vi "HEWH Dispense Schedule.vi"(0 "Core HEWH Data Input":T1={"Scan Rate Adjust"=0.0, "Draw Count"=0, "Test Patten Setup"={"Total Gallons Schedule"=[10.0, 10.0, 10.0, 10.0], "PRAT/RLT Sequence"=[{"Sequence #"=1.0, "Cycles"=35, "Mode Setting"="", "Flow Rate (GPM)"=0.0, "Temperature (F)"=0.0, "Reset Timer"=FALSE, "Use Temp Decline Method"=FALSE, "Terminate Condition"=enum."C1-Terminate Draw @ Gallon Mark", "Condition Value #1"=1.0, "UE"=FALSE, "LE"=FALSE, "Comp"=FALSE, "Fan"=FALSE, "Test End Time (Sec)"=0.0, "Purge Until Cutout"=FALSE, "Start Conditions"=enum."Heat Source Cutout", "Condition Value #2"=0.0, "Remove Power"=FALSE, "Time"=0.0, "Check Special Cond."=enum."SC1-Do Nothing", "Condition#"=enum."C1", "Draw Flags"=enum."N/A", "Data Processing Delay (FHD 15sec, UEF 5 Sec)"=0.0, "Test Complete"=FALSE, "User Setpoint"=0.0, "Tank Setpoint"=0.0}, {"Sequence #"=2.0, "Cycles"=15, "Mode Setting"="", "Flow Rate (GPM)"=0.0, "Temperature (F)"=0.0, "Reset Timer"=FALSE, "Use Temp Decline Method"=FALSE, "Terminate Condition"=enum."C1-Terminate Draw @ Gallon Mark", "Condition Value #1"=1.0, "UE"=FALSE, "LE"=FALSE, "Comp"=FALSE, "Fan"=FALSE, "Test End Time (Sec)"=0.0, "Purge Until Cutout"=FALSE, "Start Conditions"=enum."Heat Source Cutout", "Condition Value #2"=0.0, "Remove Power"=FALSE, "Time"=0.0, "Check Special Cond."=enum."SC1-Do Nothing", "Condition#"=enum."C1", "Draw Flags"=enum."N/A", "Data Processing Delay (FHD 15sec, UEF 5 Sec)"=0.0, "Test Complete"=FALSE, "User Setpoint"=0.0, "Tank Setpoint"=0.0}, {"Sequence #"=3.0, "Cycles"=35, "Mode Setting"="", "Flow Rate (GPM)"=0.0, "Temperature (F)"=0.0, "Reset Timer"=FALSE, "Use Temp Decline Method"=FALSE, "Terminate Condition"=enum."C1-Terminate Draw @ Gallon Mark", "Condition Value #1"=2.0, "UE"=FALSE, "LE"=FALSE, "Comp"=FALSE, "Fan"=FALSE, "Test End Time (Sec)"=0.0, "Purge Until Cutout"=FALSE, "Start Conditions"=enum."Heat Source Cutout", "Condition Value #2"=0.0, "Remove Power"=FALSE, "Time"=0.0, "Check Special Cond."=enum."SC1-Do Nothing", "Condition#"=enum."C1", "Draw Flags"=enum."N/A", "Data Processing Delay (FHD 15sec, UEF 5 Sec)"=0.0, "Test Complete"=FALSE, "User Setpoint"=0.0, "Tank Setpoint"=0.0}, {"Sequence #"=4.0, "Cycles"=15, "Mode Setting"="", "Flow Rate (GPM)"=0.0, "Temperature (F)"=0.0, "Reset Timer"=FALSE, "Use Temp Decline Method"=FALSE, "Terminate Condition"=enum."C1-Terminate Draw @ Gallon Mark", "Condition Value #1"=2.0, "UE"=FALSE, "LE"=FALSE, "Comp"=FALSE, "Fan"=FALSE, "Test End Time (Sec)"=0.0, "Purge Until Cutout"=FALSE, "Start Conditions"=enum."Heat Source Cutout", "Condition Value #2"=0.0, "Remove Power"=FALSE, "Time"=0.0, "Check Special Cond."=enum."SC1-Do Nothing", "Condition#"=enum."C1", "Draw Flags"=enum."N/A", "Data Processing Delay (FHD 15sec, UEF 5 Sec)"=0.0, "Test Complete"=FALSE, "User Setpoint"=0.0, "Tank Setpoint"=0.0}, {"Sequence #"=5.0, "Cycles"=35, "Mode Setting"="", "Flow Rate (GPM)"=0.0, "Temperature (F)"=0.0, "Reset Timer"=FALSE, "Use Temp Decline Method"=FALSE, "Terminate Condition"=enum."C1-Terminate Draw @ Gallon Mark", "Condition Value #1"=0.0, "UE"=FALSE, "LE"=FALSE, "Comp"=FALSE, "Fan"=FALSE, "Test End Time (Sec)"=0.0, "Purge Until Cutout"=FALSE, "Start Conditions"=enum."Heat Source Cutout", "Condition Value #2"=0.0, "Remove Power"=FALSE, "Time"=0.0, "Check Special Cond."=enum."SC1-Do Nothing", "Condition#"=enum."C1", "Draw Flags"=enum."N/A", "Data Processing Delay (FHD 15sec, UEF 5 Sec)"=0.0, "Test Complete"=FALSE, "User Setpoint"=0.0, "Tank Setpoint"=0.0}, {"Sequence #"=6.0, "Cycles"=15, "Mode Setting"="", "Flow Rate (GPM)"=0.0, "Temperature (F)"=0.0, "Reset Timer"=FALSE, "Use Temp Decline Method"=FALSE, "Terminate Condition"=enum."C1-Terminate Draw @ Gallon Mark", "Condition Value #1"=0.0, "UE"=FALSE, "LE"=FALSE, "Comp"=FALSE, "Fan"=FALSE, "Test End Time (Sec)"=0.0, "Purge Until Cutout"=FALSE, "Start Conditions"=enum."Heat Source Cutout", "Condition Value #2"=0.0, "Remove Power"=FALSE, "Time"=0.0, "Check Special Cond."=enum."SC1-Do Nothing", "Condition#"=enum."C1", "Draw Flags"=enum."N/A", "Data Processing Delay (FHD 15sec, UEF 5 Sec)"=0.0, "Test Complete"=FALSE, "User Setpoint"=0.0, "Tank Setpoint"=0.0}, {"Sequence #"=7.0, "Cycles"=35, "Mode Setting"="", "Flow Rate (GPM)"=0.0, "Temperature (F)"=0.0, "Reset Timer"=FALSE, "Use Temp Decline Method"=FALSE, "Terminate Condition"=enum."C1-Terminate Draw @ Gallon Mark", "Condition Value #1"=1.0, "UE"=FALSE, "LE"=FALSE, "Comp"=FALSE, "Fan"=FALSE, "Test End Time (Sec)"=0.0, "Purge Until Cutout"=FALSE, "Start Conditions"=enum."Heat Source Cutout", "Condition Value #2"=0.0, "Remove Power"=FALSE, "Time"=0.0, "Check Special Cond."=enum."SC1-Do Nothing", "Condition#"=enum."C1", "Draw Flags"=enum."N/A", "Data Processing Delay (FHD 15sec, UEF 5 Sec)"=0.0, "Test Complete"=FALSE, "User Setpoint"=0.0, "Tank Setpoint"=0.0}, {"Sequence #"=8.0, "Cycles"=15, "Mode Setting"="", "Flow Rate (GPM)"=0.0, "Temperature (F)"=0.0, "Reset Timer"=FALSE, "Use Temp Decline Method"=FALSE, "Terminate Condition"=enum."C1-Terminate Draw @ Gallon Mark", "Condition Value #1"=1.0, "UE"=FALSE, "LE"=FALSE, "Comp"=FALSE, "Fan"=FALSE, "Test End Time (Sec)"=0.0, "Purge Until Cutout"=FALSE, "Start Conditions"=enum."Heat Source Cutout", "Condition Value #2"=0.0, "Remove Power"=FALSE, "Time"=0.0, "Check Special Cond."=enum."SC1-Do Nothing", "Condition#"=enum."C1", "Draw Flags"=enum."N/A", "Data Processing Delay (FHD 15sec, UEF 5 Sec)"=0.0, "Test Complete"=FALSE, "User Setpoint"=0.0, "Tank Setpoint"=0.0}], "Current Sequence Index"=0}, "HEWH Specific DAQ"={"HEWH Data"={"HEWH Standard"={"Voltage (Volts)"=0.0, "Current (Amps)"=0.0, "Power (Watts)"=0.0, "WattHours (Wh)"=0.0, "TC Tree (AVG)"=0.0, "Flow Rate (GPM)"=0.0, "Gallons (Gal)"=0.0, "RTD Out (Deg F)"=0.0, "RTD In (Deg F)"=0.0, "RTD Amb (Deg F)"=0.0, "TC Down"=0.0, "UE Event Lead"=0, "LE Event Lead"=0, "TC Tree Array"=[]}, "PRAT"={"Power (Watts) A"=4192.0, "Power (Watts) B"=4192.0, "Power (Watts) C"=4192.0, "Power (Watts) D"=4192.0, "TC1"=0.0, "TC2"=0.0, "TC3"=0.0, "TC4"=0.0, "WattHours (Wh) A"=4192.0, "WattHours (Wh) B"=4192.0, "WattHours (Wh) C"=4192.0, "WattHours (Wh) D"=4192.0, "Ambient"=0.0, "Extra Temp"=0.0}, "Additional Power Data"={"Vthd"=236.2, "Frequency (Hz)"=236.2, "Apparent Power (VA)"=236.2, "Power Factor"=236.2, "Current Crest Factor"=236.2, "Voltage Crest Factor"=236.2, "Integration Time (sec)"=236.2}}, "Flow Valve % Open"=0.0, "Power State"={"UE"=FALSE, "LE"=FALSE, "COMP"=FALSE, "FANS"=FALSE}, "Power Analyzer"=enum."APLUS", "Flow Valve uA Output"=0, "Gallons Start (Gal)"=0.0}, "Test Output Data"={"PreDraw Data Table"=[], "Data Table"=[], "MW100 TC Headers"=[]}, "Calc and Calibration"={"Mean SD Var Max Min Array"=[], "Draw Statistics (DBL)"=[], "Calibration Coefficients DBL"=[], "Start Gallons"=0.0, "Starting Temp Decline"=0.0, "K-Factor (Temperature)"=0.0, "All Draw Stats"=[], "RTD Terminate Value"=0.0, "K-Factor (Flow)"=0.0, "Intellifaucet Type"="", "Thermal Stabil Array"=[], "Gas Thermal Stabil Complete"=FALSE, "Therm Reset Cmpt 1"=FALSE, "Therm Reset Cmpt 2"=FALSE, "Last Flow Rate (Therm)"=0.0, "State"=enum."State 0", "Gas Thermal Time"=0.0, "Target Rate (Thermal)"=0.0, "Thermal - Final"=[], "State5 Gal Water"=0.0, "State 5 Gal Gas"=0.0, "Intellif Open < 1"=0.0, "Intellif Open < 1.7"=0.0, "Intellif Open < 2.2"=0.0, "Intellif Open > 2.2"=0.0}, "Current Draw Time"=0.0, "LV Program"=enum."HEWH", "Station ID"=enum."A", "Current Cond"=enum."N/A", "Test Complete"=FALSE, "ANSI Rate"={"Array 1"=[], "Array 3"=[], "Array 2"=[], "Start ANSI"=FALSE, "ANSI Start Time"=0.0, "Restart ANSI"=FALSE, "15 Min ANSI Avg (BTU/hr)"=0.0, "20 Min ANSI Avg (BTU/hr)"=0.0, "25 Min ANSI Avg (BTU/hr)"=0.0, "Absolute Pressure"=0.0, "Gas Temperature"=0.0, "Volumetric Flow Rate"=0.0, "Mass Flow Rate"=0.0, "Array 4"=[], "Array 5"=[], "Gas Rate"=0.0, "15 Min Pres Avg (PSIA)"=0.0, "20 Min Pres Avg (PSIA)"=0.0, "25 Min Pres Avg (PSIA)"=0.0, "15 Min Temp Avg (°F) "=0.0, "20 Min Temp Avg (°F)"=0.0, "25 Min Temp Avg (°F)"=0.0, "15 Min Uncorrected Avg (CFH)"=0.0, "20 Min Uncorrected Avg (CFH)"=0.0, "25 Min Uncorrected Avg (CFH)"=0.0, "15 Min Corrected Avg (SCFH)"=0.0, "20 Min Corrected Avg (SCFH)"=0.0, "25 Min Corrected Avg (SCFH)"=0.0, "15 Min Complete"=FALSE, "20 Min Complete"=FALSE, "25 Min Complete"=FALSE, "Heating Value (BTU/ft³)"=0.0, "CO CO2 15 Min"=[], "CO CO2 20 Min"=[], "CO CO2 25 Min"=[], "CO CO2 Real Time"=[]}, "Gas Measurment Data"={"Absolute Pressure"=0.0, "Gauge/Diff. Pressure"=0.0, "Barometric Pressure"=0.0, "Temperature"=0.0, "Volumetric Flow"=0.0, "Mass Flow"=0.0, "Setpoint"=0.0, "Valve Drive"=0.0, "Totalizer"=0.0, "[hr]"=0.0, "[min]"=0.0, "[sec]"=0.0, "Totalizer Average Flow"=0.0, "Totalizer Peak Flow"=0.0, "Gas selected"=""}, "Module 4 Relay Status"={"INTELLIFAUCET TEMP(T)/FLOW(F) (CH 041)"=FALSE, "INTELLIFAUCET READY (CH 042)"=FALSE, "INTELLIFAUCET START (CH 043)"=FALSE, "INTELLIFAUCET STOP (CH 044)"=FALSE, "MAIN POWER RELAY (CH 047)"=FALSE, "NOT USED (CH 045)"=FALSE, "NOT USED (CH 046)"=FALSE, "PURGE VALVE RELAY (CH 048)"=FALSE, "OUTLET VALVE RELAY (CH 049)"=FALSE, "INLET VALVE RELAY (CH 050)"=FALSE, "Intellifaucet (% Open)"=0.0, "Proportioning Valve (%Open)"=0.0, "Intellifaucet Temp Setpoint (F)"=0.0}} {"Test Patten Setup"."PRAT/RLT Sequence"."Time" format="%<%H:%M:%S>t"; "Test Patten Setup"."Total Gallons Schedule" format="%.2f"}, 5 "Hide PreDraw Tab":bool, 11 "error in (no error)":errorcluster) -> (4 "Core HEWH Data Input Out":T1={"Scan Rate Adjust"=1000.0, "Draw Count"=0, "Test Patten Setup"={"Total Gallons Schedule"=[10.72, 10.72, 10.72, 10.72, 10.72, 10.72], "PRAT/RLT Sequence"=[{"Sequence #"=1.0, "Cycles"=35, "Mode Setting"="", "Flow Rate (GPM)"=0.0, "Temperature (F)"=0.0, "Reset Timer"=FALSE, "Use Temp Decline Method"=FALSE, "Terminate Condition"=enum."C1-Terminate Draw @ Gallon Mark", "Condition Value #1"=1.0, "UE"=FALSE, "LE"=FALSE, "Comp"=FALSE, "Fan"=FALSE, "Test End Time (Sec)"=0.0, "Purge Until Cutout"=FALSE, "Start Conditions"=enum."Heat Source Cutout", "Condition Value #2"=0.0, "Remove Power"=FALSE, "Time"=0.0, "Check Special Cond."=enum."SC1-Do Nothing", "Condition#"=enum."C1", "Draw Flags"=enum."N/A", "Data Processing Delay (FHD 15sec, UEF 5 Sec)"=0.0, "Test Complete"=FALSE, "User Setpoint"=0.0, "Tank Setpoint"=0.0}, {"Sequence #"=2.0, "Cycles"=15, "Mode Setting"="", "Flow Rate (GPM)"=0.0, "Temperature (F)"=0.0, "Reset Timer"=FALSE, "Use Temp Decline Method"=FALSE, "Terminate Condition"=enum."C1-Terminate Draw @ Gallon Mark", "Condition Value #1"=1.0, "UE"=FALSE, "LE"=FALSE, "Comp"=FALSE, "Fan"=FALSE, "Test End Time (Sec)"=0.0, "Purge Until Cutout"=FALSE, "Start Conditions"=enum."Heat Source Cutout", "Condition Value #2"=0.0, "Remove Power"=FALSE, "Time"=0.0, "Check Special Cond."=enum."SC1-Do Nothing", "Condition#"=enum."C1", "Draw Flags"=enum."N/A", "Data Processing Delay (FHD 15sec, UEF 5 Sec)"=0.0, "Test Complete"=FALSE, "User Setpoint"=0.0, "Tank Setpoint"=0.0}, {"Sequence #"=3.0, "Cycles"=35, "Mode Setting"="", "Flow Rate (GPM)"=0.0, "Temperature (F)"=0.0, "Reset Timer"=FALSE, "Use Temp Decline Method"=FALSE, "Terminate Condition"=enum."C1-Terminate Draw @ Gallon Mark", "Condition Value #1"=2.0, "UE"=FALSE, "LE"=FALSE, "Comp"=FALSE, "Fan"=FALSE, "Test End Time (Sec)"=0.0, "Purge Until Cutout"=FALSE, "Start Conditions"=enum."Heat Source Cutout", "Condition Value #2"=0.0, "Remove Power"=FALSE, "Time"=0.0, "Check Special Cond."=enum."SC1-Do Nothing", "Condition#"=enum."C1", "Draw Flags"=enum."N/A", "Data Processing Delay (FHD 15sec, UEF 5 Sec)"=0.0, "Test Complete"=FALSE, "User Setpoint"=0.0, "Tank Setpoint"=0.0}, {"Sequence #"=4.0, "Cycles"=15, "Mode Setting"="", "Flow Rate (GPM)"=0.0, "Temperature (F)"=0.0, "Reset Timer"=FALSE, "Use Temp Decline Method"=FALSE, "Terminate Condition"=enum."C1-Terminate Draw @ Gallon Mark", "Condition Value #1"=2.0, "UE"=FALSE, "LE"=FALSE, "Comp"=FALSE, "Fan"=FALSE, "Test End Time (Sec)"=0.0, "Purge Until Cutout"=FALSE, "Start Conditions"=enum."Heat Source Cutout", "Condition Value #2"=0.0, "Remove Power"=FALSE, "Time"=0.0, "Check Special Cond."=enum."SC1-Do Nothing", "Condition#"=enum."C1", "Draw Flags"=enum."N/A", "Data Processing Delay (FHD 15sec, UEF 5 Sec)"=0.0, "Test Complete"=FALSE, "User Setpoint"=0.0, "Tank Setpoint"=0.0}, {"Sequence #"=5.0, "Cycles"=35, "Mode Setting"="", "Flow Rate (GPM)"=0.0, "Temperature (F)"=0.0, "Reset Timer"=FALSE, "Use Temp Decline Method"=FALSE, "Terminate Condition"=enum."C1-Terminate Draw @ Gallon Mark", "Condition Value #1"=0.0, "UE"=FALSE, "LE"=FALSE, "Comp"=FALSE, "Fan"=FALSE, "Test End Time (Sec)"=0.0, "Purge Until Cutout"=FALSE, "Start Conditions"=enum."Heat Source Cutout", "Condition Value #2"=0.0, "Remove Power"=FALSE, "Time"=0.0, "Check Special Cond."=enum."SC1-Do Nothing", "Condition#"=enum."C1", "Draw Flags"=enum."N/A", "Data Processing Delay (FHD 15sec, UEF 5 Sec)"=0.0, "Test Complete"=FALSE, "User Setpoint"=0.0, "Tank Setpoint"=0.0}, {"Sequence #"=6.0, "Cycles"=15, "Mode Setting"="", "Flow Rate (GPM)"=0.0, "Temperature (F)"=0.0, "Reset Timer"=FALSE, "Use Temp Decline Method"=FALSE, "Terminate Condition"=enum."C1-Terminate Draw @ Gallon Mark", "Condition Value #1"=0.0, "UE"=FALSE, "LE"=FALSE, "Comp"=FALSE, "Fan"=FALSE, "Test End Time (Sec)"=0.0, "Purge Until Cutout"=FALSE, "Start Conditions"=enum."Heat Source Cutout", "Condition Value #2"=0.0, "Remove Power"=FALSE, "Time"=0.0, "Check Special Cond."=enum."SC1-Do Nothing", "Condition#"=enum."C1", "Draw Flags"=enum."N/A", "Data Processing Delay (FHD 15sec, UEF 5 Sec)"=0.0, "Test Complete"=FALSE, "User Setpoint"=0.0, "Tank Setpoint"=0.0}, {"Sequence #"=7.0, "Cycles"=35, "Mode Setting"="", "Flow Rate (GPM)"=0.0, "Temperature (F)"=0.0, "Reset Timer"=FALSE, "Use Temp Decline Method"=FALSE, "Terminate Condition"=enum."C1-Terminate Draw @ Gallon Mark", "Condition Value #1"=1.0, "UE"=FALSE, "LE"=FALSE, "Comp"=FALSE, "Fan"=FALSE, "Test End Time (Sec)"=0.0, "Purge Until Cutout"=FALSE, "Start Conditions"=enum."Heat Source Cutout", "Condition Value #2"=0.0, "Remove Power"=FALSE, "Time"=0.0, "Check Special Cond."=enum."SC1-Do Nothing", "Condition#"=enum."C1", "Draw Flags"=enum."N/A", "Data Processing Delay (FHD 15sec, UEF 5 Sec)"=0.0, "Test Complete"=FALSE, "User Setpoint"=0.0, "Tank Setpoint"=0.0}, {"Sequence #"=8.0, "Cycles"=15, "Mode Setting"="", "Flow Rate (GPM)"=0.0, "Temperature (F)"=0.0, "Reset Timer"=FALSE, "Use Temp Decline Method"=FALSE, "Terminate Condition"=enum."C1-Terminate Draw @ Gallon Mark", "Condition Value #1"=1.0, "UE"=FALSE, "LE"=FALSE, "Comp"=FALSE, "Fan"=FALSE, "Test End Time (Sec)"=0.0, "Purge Until Cutout"=FALSE, "Start Conditions"=enum."Heat Source Cutout", "Condition Value #2"=0.0, "Remove Power"=FALSE, "Time"=0.0, "Check Special Cond."=enum."SC1-Do Nothing", "Condition#"=enum."C1", "Draw Flags"=enum."N/A", "Data Processing Delay (FHD 15sec, UEF 5 Sec)"=0.0, "Test Complete"=FALSE, "User Setpoint"=0.0, "Tank Setpoint"=0.0}], "Current Sequence Index"=0}, "HEWH Specific DAQ"={"HEWH Data"={"HEWH Standard"={"Voltage (Volts)"=-1.0, "Current (Amps)"=-1.0, "Power (Watts)"=-1.0, "WattHours (Wh)"=-1.0, "TC Tree (AVG)"=0.0, "Flow Rate (GPM)"=0.0, "Gallons (Gal)"=0.0, "RTD Out (Deg F)"=0.0, "RTD In (Deg F)"=0.0, "RTD Amb (Deg F)"=0.0, "TC Down"=0.0, "UE Event Lead"=0, "LE Event Lead"=0, "TC Tree Array"=[]}, "PRAT"={"Power (Watts) A"=4192.0, "Power (Watts) B"=4192.0, "Power (Watts) C"=4192.0, "Power (Watts) D"=4192.0, "TC1"=0.0, "TC2"=0.0, "TC3"=0.0, "TC4"=0.0, "WattHours (Wh) A"=4192.0, "WattHours (Wh) B"=4192.0, "WattHours (Wh) C"=4192.0, "WattHours (Wh) D"=4192.0, "Ambient"=0.0, "Extra Temp"=0.0}, "Additional Power Data"={"Vthd"=236.2, "Frequency (Hz)"=236.2, "Apparent Power (VA)"=236.2, "Power Factor"=236.2, "Current Crest Factor"=236.2, "Voltage Crest Factor"=236.2, "Integration Time (sec)"=236.2}}, "Flow Valve % Open"=0.0, "Power State"={"UE"=FALSE, "LE"=FALSE, "COMP"=FALSE, "FANS"=FALSE}, "Power Analyzer"=enum."APLUS", "Flow Valve uA Output"=0, "Gallons Start (Gal)"=0.0}, "Test Output Data"={"PreDraw Data Table"=[], "Data Table"=[], "MW100 TC Headers"=[]}, "Calc and Calibration"={"Mean SD Var Max Min Array"=[], "Draw Statistics (DBL)"=[], "Calibration Coefficients DBL"=[], "Start Gallons"=0.0, "Starting Temp Decline"=1000.0, "K-Factor (Temperature)"=0.0, "All Draw Stats"=[], "RTD Terminate Value"=0.0, "K-Factor (Flow)"=0.0, "Intellifaucet Type"="", "Thermal Stabil Array"=[], "Gas Thermal Stabil Complete"=FALSE, "Therm Reset Cmpt 1"=FALSE, "Therm Reset Cmpt 2"=FALSE, "Last Flow Rate (Therm)"=0.0, "State"=enum."State 0", "Gas Thermal Time"=0.0, "Target Rate (Thermal)"=0.0, "Thermal - Final"=[], "State5 Gal Water"=0.0, "State 5 Gal Gas"=0.0, "Intellif Open < 1"=0.0, "Intellif Open < 1.7"=0.0, "Intellif Open < 2.2"=0.0, "Intellif Open > 2.2"=0.0}, "Current Draw Time"=0.0, "LV Program"=enum."HEWH", "Station ID"=enum."A", "Current Cond"=enum."N/A", "Test Complete"=FALSE, "ANSI Rate"={"Array 1"=[], "Array 3"=[], "Array 2"=[], "Start ANSI"=FALSE, "ANSI Start Time"=0.0, "Restart ANSI"=FALSE, "15 Min ANSI Avg (BTU/hr)"=0.0, "20 Min ANSI Avg (BTU/hr)"=0.0, "25 Min ANSI Avg (BTU/hr)"=0.0, "Absolute Pressure"=0.0, "Gas Temperature"=0.0, "Volumetric Flow Rate"=0.0, "Mass Flow Rate"=0.0, "Array 4"=[], "Array 5"=[], "Gas Rate"=0.0, "15 Min Pres Avg (PSIA)"=0.0, "20 Min Pres Avg (PSIA)"=0.0, "25 Min Pres Avg (PSIA)"=0.0, "15 Min Temp Avg (°F) "=0.0, "20 Min Temp Avg (°F)"=0.0, "25 Min Temp Avg (°F)"=0.0, "15 Min Uncorrected Avg (CFH)"=0.0, "20 Min Uncorrected Avg (CFH)"=0.0, "25 Min Uncorrected Avg (CFH)"=0.0, "15 Min Corrected Avg (SCFH)"=0.0, "20 Min Corrected Avg (SCFH)"=0.0, "25 Min Corrected Avg (SCFH)"=0.0, "15 Min Complete"=FALSE, "20 Min Complete"=FALSE, "25 Min Complete"=FALSE, "Heating Value (BTU/ft³)"=0.0, "CO CO2 15 Min"=[], "CO CO2 20 Min"=[], "CO CO2 25 Min"=[], "CO CO2 Real Time"=[]}, "Gas Measurment Data"={"Absolute Pressure"=0.0, "Gauge/Diff. Pressure"=0.0, "Barometric Pressure"=0.0, "Temperature"=0.0, "Volumetric Flow"=0.0, "Mass Flow"=0.0, "Setpoint"=0.0, "Valve Drive"=0.0, "Totalizer"=0.0, "[hr]"=0.0, "[min]"=0.0, "[sec]"=0.0, "Totalizer Average Flow"=0.0, "Totalizer Peak Flow"=0.0, "Gas selected"=""}, "Module 4 Relay Status"={"INTELLIFAUCET TEMP(T)/FLOW(F) (CH 041)"=FALSE, "INTELLIFAUCET READY (CH 042)"=FALSE, "INTELLIFAUCET START (CH 043)"=FALSE, "INTELLIFAUCET STOP (CH 044)"=FALSE, "MAIN POWER RELAY (CH 047)"=FALSE, "NOT USED (CH 045)"=FALSE, "NOT USED (CH 046)"=FALSE, "PURGE VALVE RELAY (CH 048)"=FALSE, "OUTLET VALVE RELAY (CH 049)"=FALSE, "INLET VALVE RELAY (CH 050)"=FALSE, "Intellifaucet (% Open)"=0.0, "Proportioning Valve (%Open)"=0.0, "Intellifaucet Temp Setpoint (F)"=0.0}} {"Test Patten Setup"."PRAT/RLT Sequence"."Time" format="%<%H:%M:%S>t"; "Test Patten Setup"."Total Gallons Schedule" format="%.2f"}, 15 "error out":errorcluster)   [LabVIEW 2019]
uses:
  Type Definitions/HEWH PreDraw.ctl
  Type Definitions/HEWH Draw Pattern Setup.ctl
  Type Definitions/HEWH Power Elements.ctl
  Type Definitions/HEWH Power Data.ctl
  Utility/Type Definitions/UTILITY Power Analyzer.ctl
  Type Definitions/HEWH Output Information.ctl
  Utility/Save File/File Setup (Public)/Type Definition/Save File DOE LabView Program.ctl
  Utility/Save File/File Setup.lvlib
  Custom Instrument Control/MW100/Type Definitions/Station ID Selector.ctl
  Utility/Save File/File Setup (Public)/Type Definition/Save File HEWH Heating Control Mode.ctl
  Type Definitions/PRAT Test.ctl
  Type Definitions/HEWH Calc and Calibration.ctl
  Draw Water Specific/Type Definitions/Terminate Draw Conditions.ctl
  Type Definitions/HEWH Start Conditions.ctl
  Type Definitions/HEWH Specific DAQ.ctl
  Draw Water Specific/Type Definitions/Check Special Condtions.ctl
  Type Definitions/HEWH Draw Flag ENUM.ctl
  Draw Water Specific/Type Definitions/HEWH Special Condition Check.ctl
  Range/Type Definitions/RANGE ANSI Rate.ctl
  Drivers/Alicat Gas Meter Driver/Sub-VIs/Data Cluster.ctl
  Custom Instrument Control/MW100/Type Definitions/HEWH Module 4 Relay Status.ctl
panel:
  in  "Tab Control":enum32{"Input", "Diagnostics"}(tab)
  out "Display and Exit":bool
  out "PreDraw\nPattern":dbl[][](array[numeric])
  in  "Draw Pattern Setup Tab":T20(tab)
  in  "Populate Older":bool
  in  "Populate Low Usage":bool
  in  "Populate Medium Usage":bool
  in  "Populate High Usage":bool
  in  "Pattern Setup":dbl[][](array[numeric])
  in  "High Usage":bool
  in  "Medium Usage":bool
  in  "Low Usage":bool
  in  "Older":bool
  out "Description":string="Pre-Draw Setup"
  out "Description 1":string="Pre-Draw Setup"
  in  "Total Gallons (1)":dbl=10.72
  in  "Flow Rate (GPM 1)":dbl=3.0
  in  "Incoming Water Temperature (1)":dbl=58.0
  out "Description 4":string="OR"
  in  "Any Heat (1)":bool
  in  "Any Heat (2)":bool
  in  "Any Heat (3)":bool
  out "Description 2":string="Pre-Draw Setup"
  in  "Total Gallons (2)":dbl=10.72
  in  "Flow Rate (GPM 2)":dbl=3.0
  in  "Incoming Water Temperature (2)":dbl=58.0
  out "Description 3":string="Pre-Draw Setup"
  in  "Total Gallons (3)":dbl=10.72
  in  "Flow Rate (GPM 3)":dbl=3.0
  in  "Incoming Water Temperature (3)":dbl=58.0
  out "Description 5":string="OR"
  out "Description 6":string="OR"
  in  "PreDraw Enum":T21=enum.""
  in  "stop":bool
  # "Draw Patten Setup"
  # "Totalizer Timer"
  # "Draw Pattern Setup (24 Hour)"
  # "Totalizer Timer"
  # "Draw Pattern Setup (24 Hour)"
  # "Dispense Times\n(Hour)"
  # "Dispense Times\n(Minutes)"
  # "Dispense Times\n(Seconds)"
  # "Total Gallons"
  # "Flow Rate\n(GPM)"
  # "Incoming Water\n Temperature"
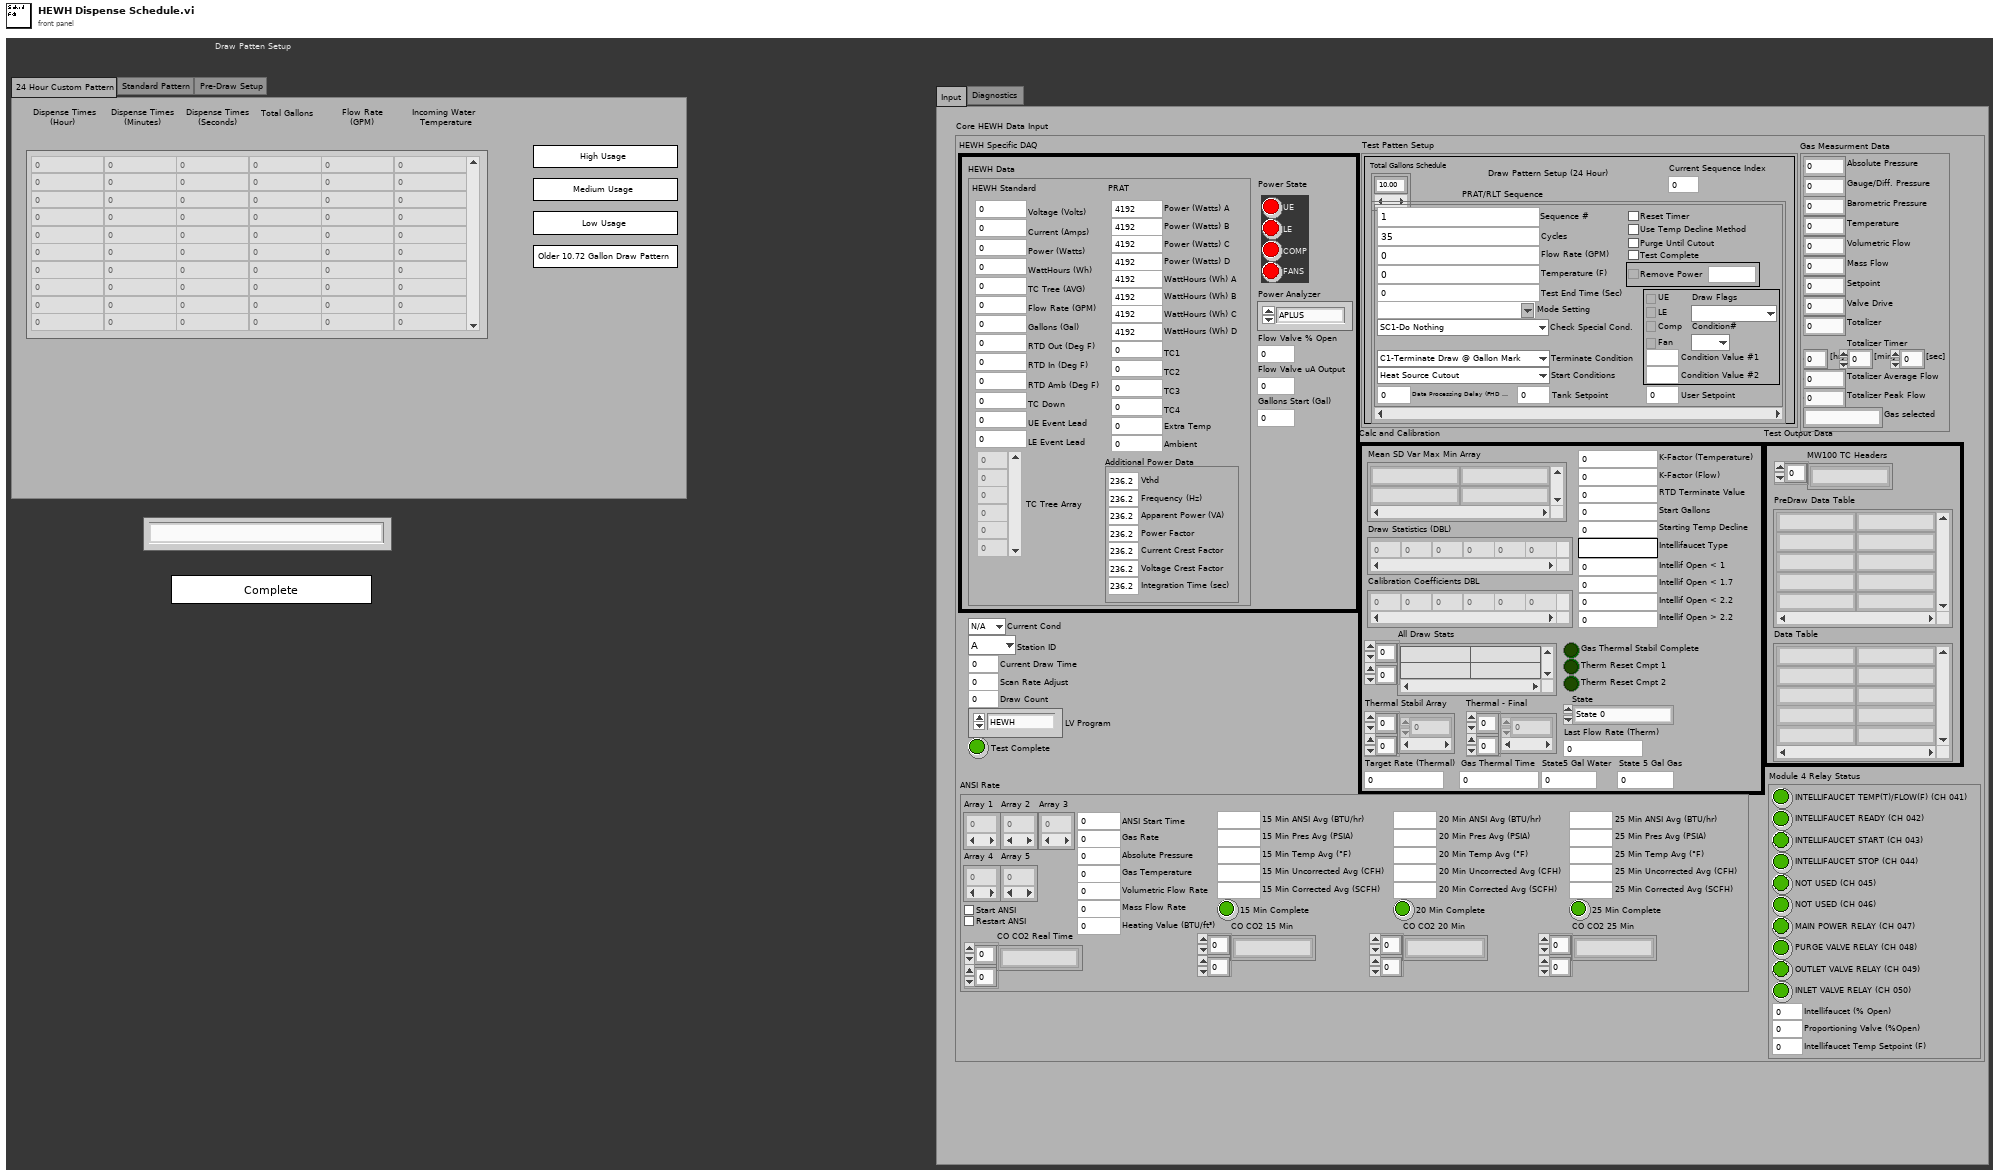
[diagram p1: front panel]
types:
  T1 = typedef "HEWH Output Information.ctl" = cluster{"Scan Rate Adjust":dbl, "Draw Count":i32, "Test Patten Setup":T2, "HEWH Specific DAQ":T10, "Test Output Data":cluster{"PreDraw Data Table":string[][], "Data Table":string[][], "MW100 TC Headers":string[]}, "Calc and Calibration":T14, "Current Draw Time":dbl, "LV Program":T15, "Station ID":T16, "Current Cond":T8, "Test Complete":bool, "ANSI Rate":T17, "Gas Measurment Data":T18, "Module 4 Relay Status":T19}
  T2 = typedef "HEWH Draw Pattern Setup.ctl" = cluster{"Total Gallons Schedule":dbl[], "PRAT/RLT Sequence":T3[], "Current Sequence Index":i32}
  T3 = typedef "PRAT Test.ctl" = cluster{"Sequence #":dbl, "Cycles":i32, "Mode Setting":T4, "Flow Rate (GPM)":dbl, "Temperature (F)":dbl, "Reset Timer":bool, "Use Temp Decline Method":bool, "Terminate Condition":T5, "Condition Value #1":dbl, "UE":bool, "LE":bool, "Comp":bool, "Fan":bool, "Test End Time (Sec)":dbl, "Purge Until Cutout":bool, "Start Conditions":T6, "Condition Value #2":dbl, "Remove Power":bool, "Time":dbl, "Check Special Cond.":T7, "Condition#":T8, "Draw Flags":T9, "Data Processing Delay (FHD 15sec, UEF 5 Sec)":dbl, "Test Complete":bool, "User Setpoint":dbl, "Tank Setpoint":dbl}
  T4 = typedef "File Setup.lvlib/Save File HEWH Heating Control Mode.ctl" = string
  T5 = typedef "Terminate Draw Conditions.ctl" = enum16{"C1-Terminate Draw @ Gallon Mark", "C2-Special Last Draw (HU Test)", "C3-RTD Out <=", "C4-Mean Tank Temp <=", "C5-Decrease RTD Out (Deg F)", "C6-Time (Seconds)", "C7-Until Any Heat Source", "C8-Specific Heat Source", "C9-Do Nothing", "C10-Inlet Outlet RTD Temp Delta"}
  T6 = typedef "HEWH Start Conditions.ctl" = enum16{"Heat Source Cutout", "At Time (Seconds)", "Every X (Seconds)", "T2 >= X° Below Setpoint", "Seconds From Complete", "Wait for LE & Comp Cutout", "Wait for Comp Cutout", "Wait for LE Cutout", "Wait for UE Cutout", "Start Immediately"}
  T7 = typedef "Check Special Condtions.ctl" = enum16{"SC1-Do Nothing", "SC2-Check Heat Source (On-C2/Off-C1)", "SC3-Check Skip Condition", "SC4-Check Heat Source ON/Fail", "SC5-Keep Draw Valves Open", "SC6-Skip Purge"}
  T8 = typedef "HEWH Special Condition Check.ctl" = enum16{"N/A", "C1", "C2", "Reset/Fail", "Skip Draw Sequence"}
  T9 = typedef "HEWH Draw Flag ENUM.ctl" = enum16{"N/A", "None(0)", "Sml(1)", "Med(2)", "SmlMed(3)", "Lrg(4)", "SmlLrg(5)", "MedLrg(6)", "SmlMedLrg(7)"}
  T10 = typedef "HEWH Specific DAQ.ctl" = cluster{"HEWH Data":T11, "Flow Valve % Open":dbl, "Power State":T12, "Power Analyzer":T13, "Flow Valve uA Output":i32, "Gallons Start (Gal)":dbl}
  T11 = typedef "HEWH Power Data.ctl" = cluster{"HEWH Standard":cluster{"Voltage (Volts)":dbl, "Current (Amps)":dbl, "Power (Watts)":dbl, "WattHours (Wh)":dbl, "TC Tree (AVG)":dbl, "Flow Rate (GPM)":dbl, "Gallons (Gal)":dbl, "RTD Out (Deg F)":dbl, "RTD In (Deg F)":dbl, "RTD Amb (Deg F)":dbl, "TC Down":dbl, "UE Event Lead":i32, "LE Event Lead":i32, "TC Tree Array":dbl[]}, "PRAT":cluster{"Power (Watts) A":dbl, "Power (Watts) B":dbl, "Power (Watts) C":dbl, "Power (Watts) D":dbl, "TC1":dbl, "TC2":dbl, "TC3":dbl, "TC4":dbl, "WattHours (Wh) A":dbl, "WattHours (Wh) B":dbl, "WattHours (Wh) C":dbl, "WattHours (Wh) D":dbl, "Ambient":dbl, "Extra Temp":dbl}, "Additional Power Data":cluster{"Vthd":dbl, "Frequency (Hz)":dbl, "Apparent Power (VA)":dbl, "Power Factor":dbl, "Current Crest Factor":dbl, "Voltage Crest Factor":dbl, "Integration Time (sec)":dbl}}
  T12 = typedef "HEWH Power Elements.ctl" = cluster{"UE":bool, "LE":bool, "COMP":bool, "FANS":bool}
  T13 = typedef "UTILITY Power Analyzer.ctl" = enum16{"", "APLUS", "WT210", "WT500", "WT300", "OSI", "Debug", "WT230", "WT300_1", "WT300_2"}
  T14 = typedef "HEWH Calc and Calibration.ctl" = cluster{"Mean SD Var Max Min Array":string[][], "Draw Statistics (DBL)":dbl[][], "Calibration Coefficients DBL":dbl[][], "Start Gallons":dbl, "Starting Temp Decline":dbl, "K-Factor (Temperature)":dbl, "All Draw Stats":string[][], "RTD Terminate Value":dbl, "K-Factor (Flow)":dbl, "Intellifaucet Type":string, "Thermal Stabil Array":dbl[][], "Gas Thermal Stabil Complete":bool, "Therm Reset Cmpt 1":bool, "Therm Reset Cmpt 2":bool, "Last Flow Rate (Therm)":dbl, "State":enum16{"State 0", "State 1", "State 2", "State 3", "State 4", "State 5", "State 6"}, "Gas Thermal Time":dbl, "Target Rate (Thermal)":dbl, "Thermal - Final":dbl[][], "State5 Gal Water":dbl, "State 5 Gal Gas":dbl, "Intellif Open < 1":dbl, "Intellif Open < 1.7":dbl, "Intellif Open < 2.2":dbl, "Intellif Open > 2.2":dbl}
  T15 = typedef "File Setup.lvlib/Save File DOE LabView Program.ctl" = enum16{"No Name Found", "DOE Stand", "Dishwasher Kitchen", "Portable Stand", "HEWH", "Dryer", "Dryer WILT", "HCC", "PRAT", "HEWH RLT", "Refrigeration", "Gas Water Heater"}
  T16 = typedef "Station ID Selector.ctl" = enum16{"", "A", "B", "C", "D", "Global"}
  T17 = typedef "RANGE ANSI Rate.ctl" = cluster{"Array 1":dbl[], "Array 3":dbl[], "Array 2":dbl[], "Start ANSI":bool, "ANSI Start Time":dbl, "Restart ANSI":bool, "15 Min ANSI Avg (BTU/hr)":dbl, "20 Min ANSI Avg (BTU/hr)":dbl, "25 Min ANSI Avg (BTU/hr)":dbl, "Absolute Pressure":dbl, "Gas Temperature":dbl, "Volumetric Flow Rate":dbl, "Mass Flow Rate":dbl, "Array 4":dbl[], "Array 5":dbl[], "Gas Rate":dbl, "15 Min Pres Avg (PSIA)":dbl, "20 Min Pres Avg (PSIA)":dbl, "25 Min Pres Avg (PSIA)":dbl, "15 Min Temp Avg (°F) ":dbl, "20 Min Temp Avg (°F)":dbl, "25 Min Temp Avg (°F)":dbl, "15 Min Uncorrected Avg (CFH)":dbl, "20 Min Uncorrected Avg (CFH)":dbl, "25 Min Uncorrected Avg (CFH)":dbl, "15 Min Corrected Avg (SCFH)":dbl, "20 Min Corrected Avg (SCFH)":dbl, "25 Min Corrected Avg (SCFH)":dbl, "15 Min Complete":bool, "20 Min Complete":bool, "25 Min Complete":bool, "Heating Value (BTU/ft³)":dbl, "CO CO2 15 Min":string[][], "CO CO2 20 Min":string[][], "CO CO2 25 Min":string[][], "CO CO2 Real Time":string[][]}
  T18 = typedef "Data Cluster.ctl" = cluster{"Absolute Pressure":dbl, "Gauge/Diff. Pressure":dbl, "Barometric Pressure":dbl, "Temperature":dbl, "Volumetric Flow":dbl, "Mass Flow":dbl, "Setpoint":dbl, "Valve Drive":dbl, "Totalizer":dbl, "[hr]":dbl, "[min]":dbl, "[sec]":dbl, "Totalizer Average Flow":dbl, "Totalizer Peak Flow":dbl, "Gas selected":string}
  T19 = typedef "HEWH Module 4 Relay Status.ctl" = cluster{"INTELLIFAUCET TEMP(T)/FLOW(F) (CH 041)":bool, "INTELLIFAUCET READY (CH 042)":bool, "INTELLIFAUCET START (CH 043)":bool, "INTELLIFAUCET STOP (CH 044)":bool, "MAIN POWER RELAY (CH 047)":bool, "NOT USED (CH 045)":bool, "NOT USED (CH 046)":bool, "PURGE VALVE RELAY (CH 048)":bool, "OUTLET VALVE RELAY (CH 049)":bool, "INLET VALVE RELAY (CH 050)":bool, "Intellifaucet (% Open)":dbl, "Proportioning Valve (%Open)":dbl, "Intellifaucet Temp Setpoint (F)":dbl}
  T20 = enum32{"24 Hour Custom Pattern", "Standard Pattern", "Pre-Draw Setup"}
  T21 = typedef "HEWH PreDraw.ctl" = enum16{"Zero Pre-Draws", "One Pre- Draws", "Two Pre-Draws", "Three Pre-Draws", ""}
  T22 = enum32{"invalid app kind", "Development System", "Run Time System", "Student Edition", "Embedded LabVIEW", "Evaluation", "Custom"}
  T23 = enum32{"Invalid", "Standard", "Closed", "Hidden", "Minimized", "Maximized"}
  T24 = cluster{"Core":cluster{"Current VI Reference":refnum<vi>, "Close Panel on Exit?":bool}, "Pattern Setup":dbl[][], "Core HEWH Data Input":T1, "PreDraw Enum":T21, "Any Heat (1)":bool, "Any Heat (2)":bool, "Any Heat (3)":bool}
  T25 = cluster{"Current VI Reference":refnum<vi>, "Close Panel on Exit?":bool}
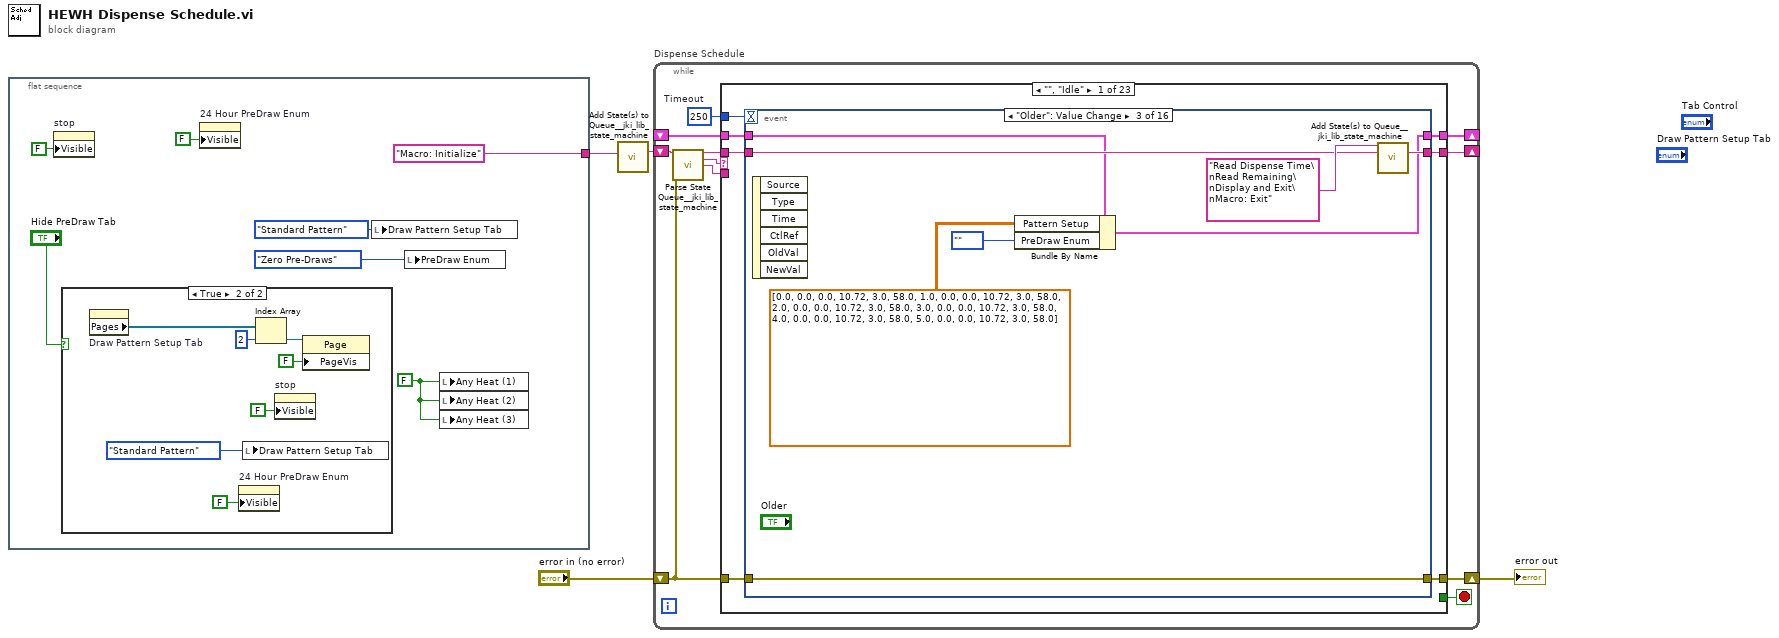
[diagram p0: block diagram]
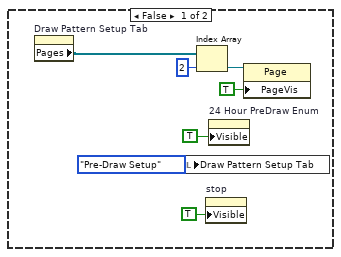
[diagram p2: hidden frame]
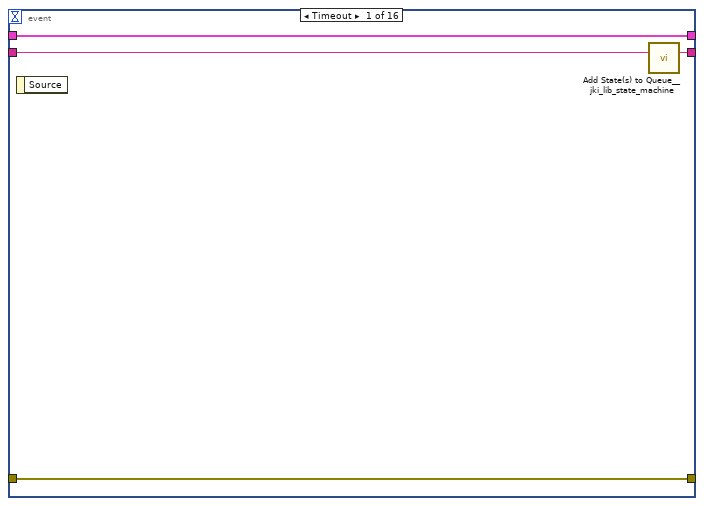
[diagram p3: hidden frame]
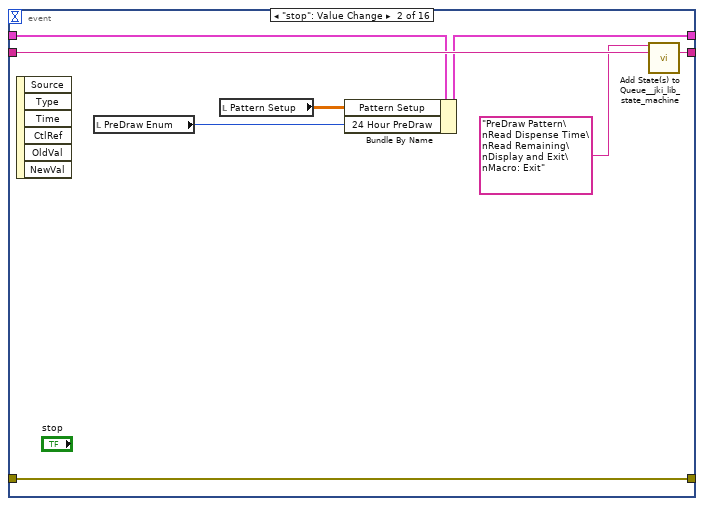
[diagram p4: hidden frame]
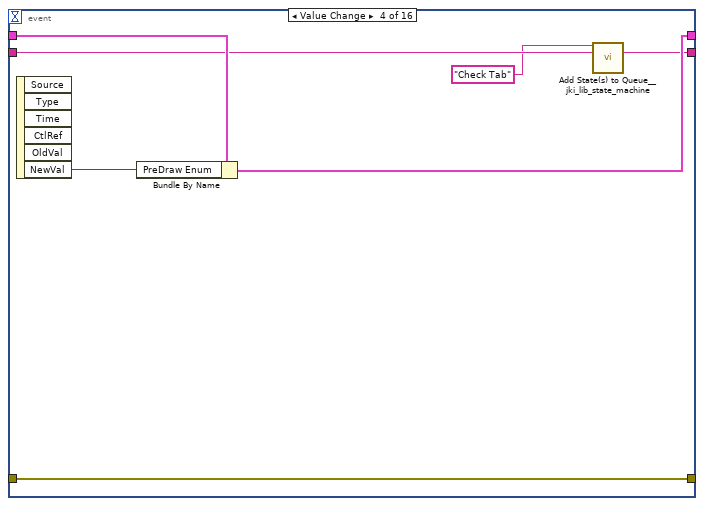
[diagram p5: hidden frame]
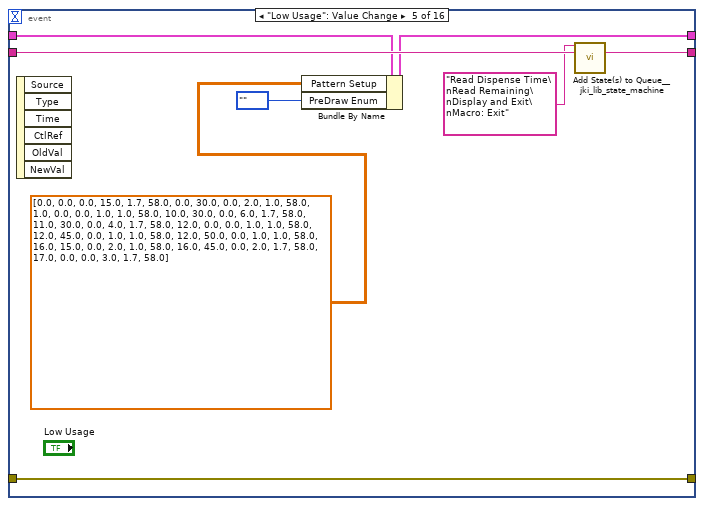
[diagram p6: hidden frame]
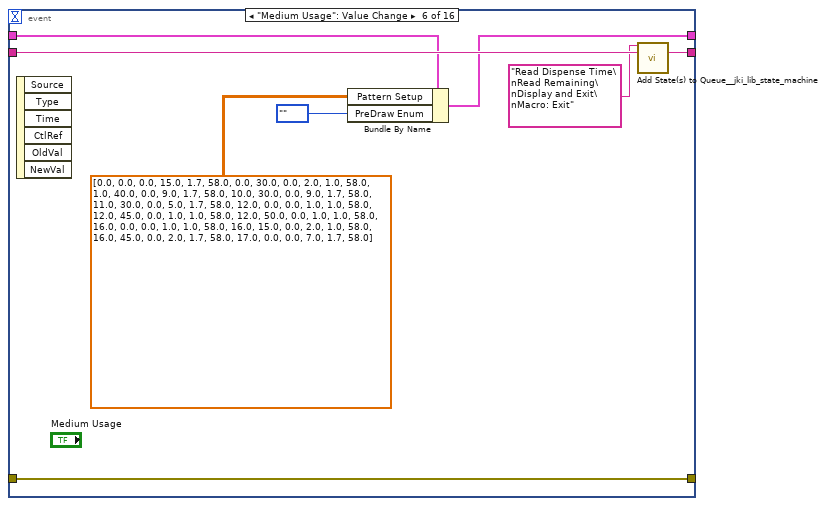
[diagram p7: hidden frame]
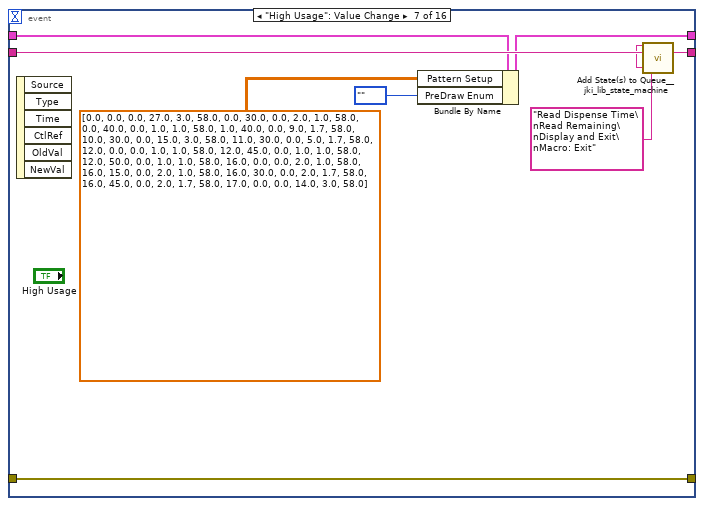
[diagram p8: hidden frame]
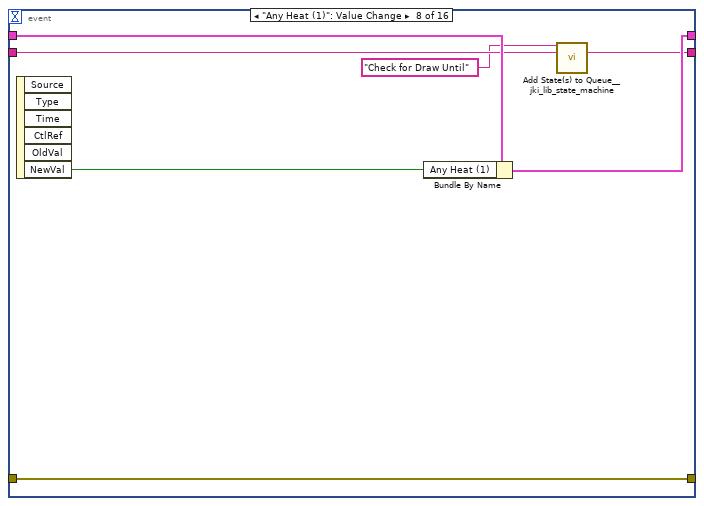
[diagram p9: hidden frame]
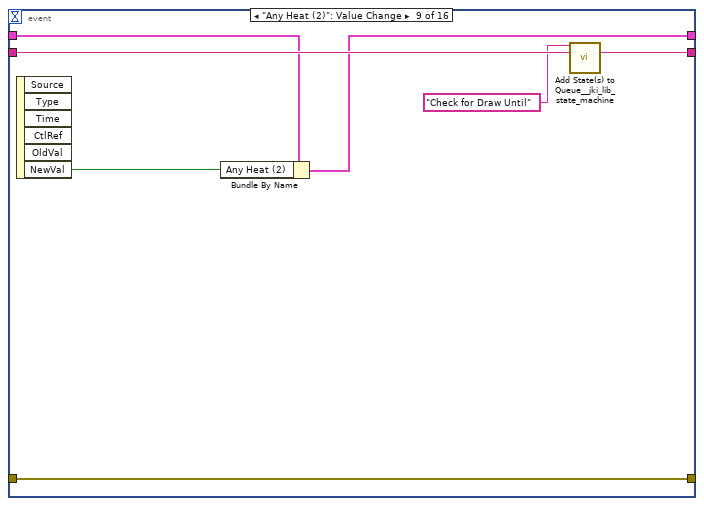
[diagram p10: hidden frame]
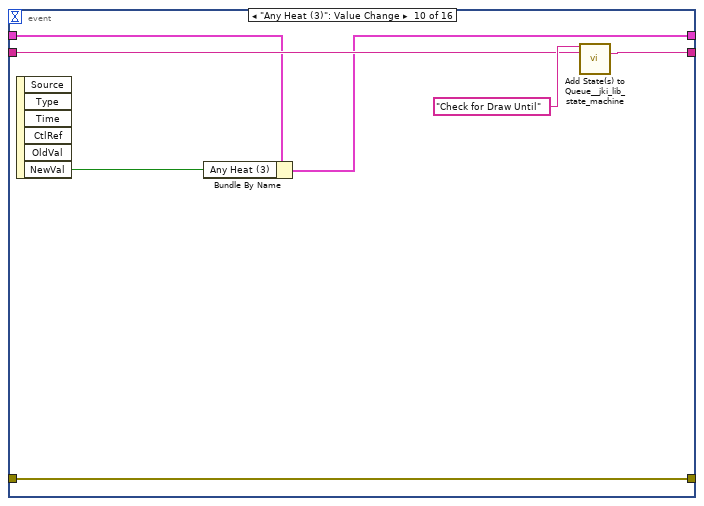
[diagram p11: hidden frame]
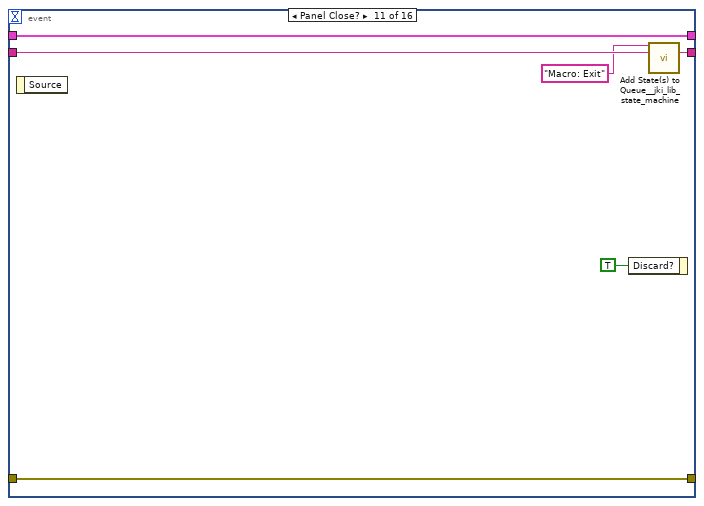
[diagram p12: hidden frame]
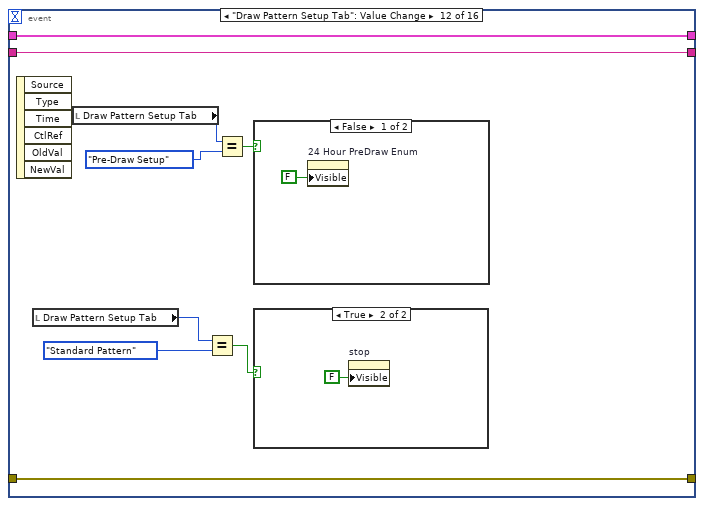
[diagram p13: hidden frame]
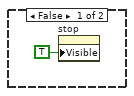
[diagram p14: hidden frame]
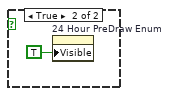
[diagram p15: hidden frame]
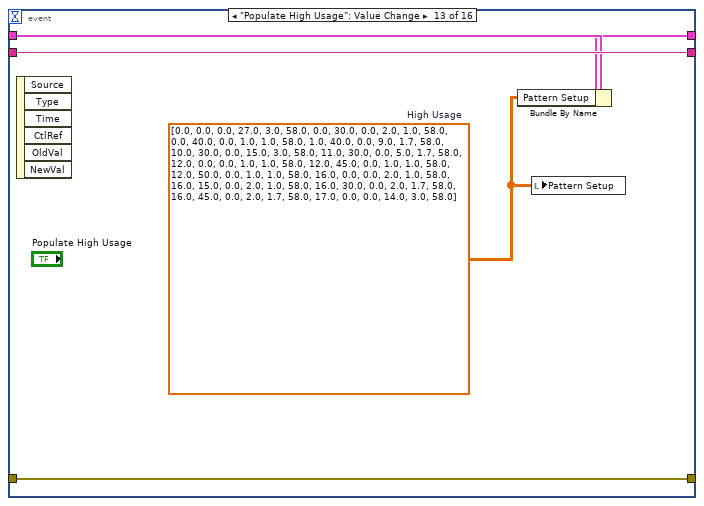
[diagram p16: hidden frame]
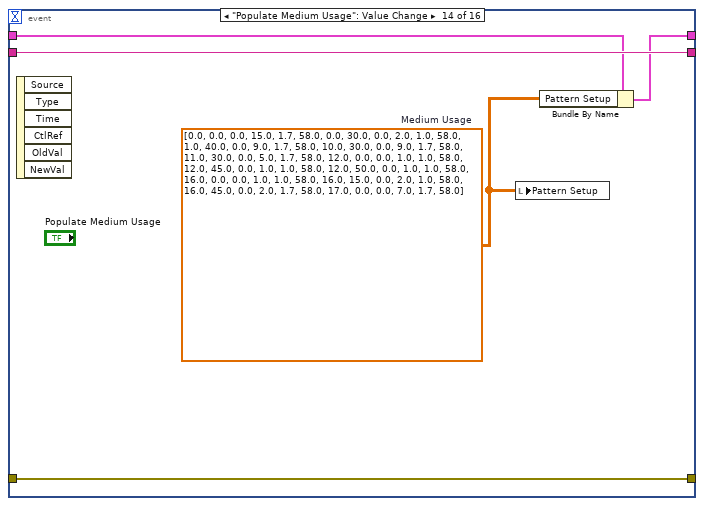
[diagram p17: hidden frame]
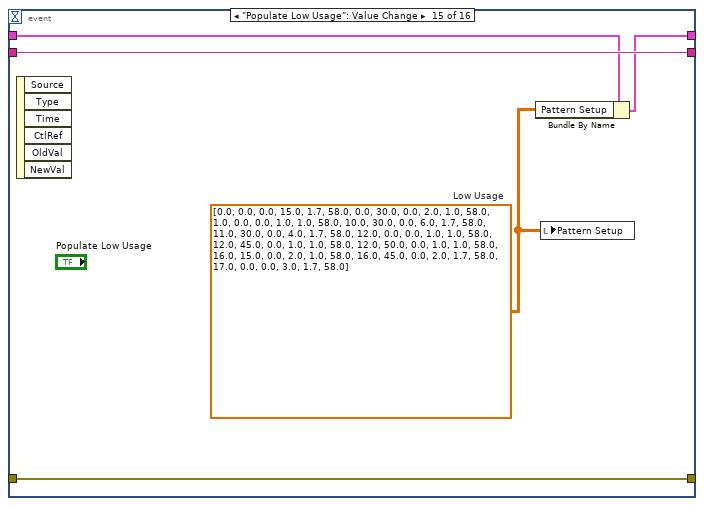
[diagram p18: hidden frame]
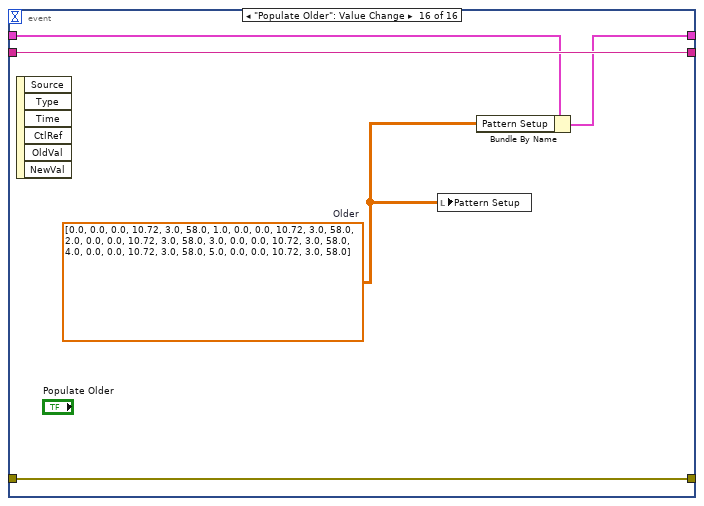
[diagram p19: hidden frame]
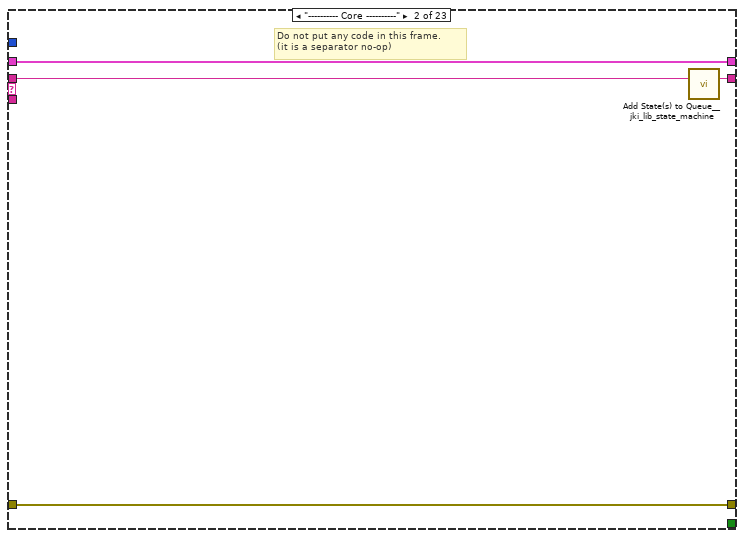
[diagram p20: hidden frame]
diagram:
  n1 = flat-sequence {
    tunnel: ["Macro: Initialize"] -> w3
    frame #0 {
      w9 = FALSE
      n2 = property on="stop" class="Bool"("Visible"=FALSE) -> ()  [unwired: 2 in, 2 out]
      n3 = case shown="True" "Hide PreDraw Tab" {
        frame False {
          n4 = property on="Draw Pattern Setup Tab" class="TabCtl (strict)"() -> ("Pages"=w12:refnum<vi>[])  [unwired: 2 in, 2 out]
          n5 = local write "Draw Pattern Setup Tab"(T20."Pre-Draw Setup" ("Draw Pattern Setup")) -> ()
          n6 = Index Array(array=w12, index=2) -> (element=w17:refnum<vi>)
          n7 = property on="stop" class="Bool"("Visible"=TRUE) -> ()  [unwired: 2 in, 2 out]
          n8 = property on="24 Hour PreDraw Enum" class="Enum (strict)"("Visible"=TRUE) -> ()  [unwired: 2 in, 2 out]
          n9 = property class="Page"(reference=w17, "PageVis"=TRUE ("Page Visible")) -> ()  [unwired: 1 in, 2 out]
        }
        frame True {
          n10 = property on="Draw Pattern Setup Tab" class="TabCtl (strict)"() -> ("Pages"=w19:refnum<vi>[])  [unwired: 2 in, 2 out]
          n11 = property on="24 Hour PreDraw Enum" class="Enum (strict)"("Visible"=FALSE) -> ()  [unwired: 2 in, 2 out]
          n12 = local write "Draw Pattern Setup Tab"(T20."Standard Pattern" ("Draw Pattern Setup")) -> ()
          n13 = Index Array(array=w19, index=2) -> (element=w24:refnum<vi>)
          n14 = property on="stop" class="Bool"("Visible"=FALSE) -> ()  [unwired: 2 in, 2 out]
          n15 = property class="Page"(reference=w24, "PageVis"=FALSE ("Page Visible")) -> ()  [unwired: 1 in, 2 out]
        }
      }
      n16 = property on="24 Hour PreDraw Enum" class="Enum (strict)"("Visible"=FALSE) -> ()  [unwired: 2 in, 2 out]
      n17 = local write "Draw Pattern Setup Tab"(T20."Standard Pattern" ("Draw Pattern Setup")) -> ()
      n18 = local write "PreDraw Enum"(HEWH_PreDraw."Zero Pre-Draws" ("24 Hour PreDraw")) -> ()
      n19 = local write "Any Heat (1)"(w9) -> ()
      n20 = local write "Any Heat (2)"(w9) -> ()
      n21 = local write "Any Heat (3)"(w9) -> ()
    }
  }
  n22 = call <vilib>:"Add State(s) to Queue__jki_lib_state_machine.vi"("State(s) in (\"\")"=w3) -> ("States Out"=w4:string)  [unwired: 14 in]
  n23 = while "Dispense Schedule" {
    shift-right: [w29] -> _
    shift-left: _ -> [w28]
    shift-right: [w32] -> w1
    shift-left: "error in (no error)" -> [w26]
    shift-right: [w31] -> _
    shift-left: w4 -> [w33]
    stop <- w30 stop-if-true
    w27 = 250  # Timeout
    n24 = call <vilib>:"Parse State Queue__jki_lib_state_machine.vi"("State Queue"=w33, "Error In (no error)"=w26) -> ("Remaining States"=w35:string, "Current State"=w36:string, "Arguments"=w34:string)  [unwired: 11 in]
    n25 = case shown="\"\", \"Idle\"" w36 {
      selector: w36 -> [_ _ w159 _ _ _ _ _ _ _ _ _ _ _ _ _ _ _ _ _ _ _ _]
      tunnel: w35 -> [w43 w158 w163 w181 w187 w192 w196 w207 w213 w217 w226 w232 w243 w269 w274 w284 w288 w293 w331 w374 w393 w409 w450]
      tunnel: w34 -> [_ _ _ _ _ _ _ _ _ _ _ w227 w237 _ _ _ _ _ _ _ _ _ _]
      tunnel: w28 -> [w41 w155 w161 w172 w184 w190 w193 _ w208 w214 w224 w230 w239 w266 w270 w281 w285 w290 w328 w364 w389 w407 w448]
      tunnel: [w40 w156 w165 w178 errorcluster {"status"=FALSE, "code"=0, "source"=""} ("error out") w189 w194 w204 w209 w215 w223 w228 w240 w267 w272 w282 w286 w291 w329 w372 w391 w404 w449] -> w32
      tunnel: w26 -> [w39 w156 w164 w178 w183 w189 w194 w204 w210 w215 w223 w229 w241 w267 w272 w282 w286 w291 w329 w372 w391 w404 w449]
      tunnel: [w42 w157 w162 w180 w186 w191 w195 w206 w212 w216 w225 w231 w242 w268 w273 w283 w287 w292 w330 w373 w392 w410 w451] -> w31
      tunnel: [_ _ _ _ _ TRUE _ _ _ _ _ _ _ _ _ _ _ _ _ _ _ _ _] -> w30
      tunnel: [w38 w155 w161 w179 w184 w190 w193 w205 w208 w214 w224 w230 w239 w266 w270 w281 w285 w290 w328 w363 w388 w408 w448] -> w29
      tunnel: w27 -> [w37 _ _ _ _ _ _ _ _ _ _ _ _ _ _ _ _ _ _ _ _ _ _]
      frame "", "Idle" {
        n26 = event shown="[2] \"Older\": Value Change" {
          selector: _ -> [_ _ _ _ _ _ _ _ _ _ _ _ _ _ _ _]
          dyn-events: _ -> [_ _ _ _ _ _ _ _ _ _ _ _ _ _ _ _]
          timeout: w37 -> [_ _ _ _ _ _ _ _ _ _ _ _ _ _ _ _]
          tunnel: w43 -> [w47 w55 w61 w66 w77 w85 w93 w97 w107 w113 w121 w129 w139 w144 w149 w154]
          tunnel: [w46 w54 w60 w65 w76 w84 w92 w96 w106 w114 w120 w129 w139 w144 w149 w154] -> w42
          tunnel: w41 -> [w44 w51 w59 w69 w74 w82 w90 w100 w104 w111 w118 w130 w138 w143 w148 w153]
          tunnel: [w45 w53 w63 w70 w78 w86 w94 w101 w108 w112 w119 w128 w135 w140 w145 w151] -> w40
          tunnel: w39 -> [w45 w53 w63 w70 w78 w86 w94 w101 w108 w112 w119 w128 w135 w140 w145 w151]
          tunnel: [w44 w50 w58 w68 w73 w81 w89 w99 w103 w110 w118 w130 w137 w142 w147 w152] -> w38
          event Timeout {
            n27 = event-data() -> ()  [unwired: 1 in, 1 out]
            n28 = call <vilib>:"Add State(s) to Queue__jki_lib_state_machine.vi"("State(s) in (\"\")"=w47) -> ("States Out"=w46:string)  [unwired: 14 in]
          }
          event "stop": Value Change {
            n29 = event-data() -> ()  [unwired: 1 in, 6 out]
            n30 = local read "PreDraw Enum"() -> (w48:T21)
            n31 = local read "Pattern Setup"() -> (w49:dbl[][])
            n32 = Bundle By Name(cluster=w51, "Pattern Setup"=w49, "24 Hour PreDraw"=w48) -> (w50:T24)
            n33 = call <vilib>:"Add State(s) to Queue__jki_lib_state_machine.vi"("State(s) in Front (\"\")"="PreDraw Pattern\nRead Dispense Time\nRead Remaining\nDisplay and Exit\nMacro: Exit", "State(s) in (\"\")"=w55) -> ("States Out"=w54:string)  [unwired: 13 in]
          }
          event "Older": Value Change {
            n34 = event-data() -> ()  [unwired: 1 in, 6 out]
            n35 = Bundle By Name(cluster=w59, "Pattern Setup"=dbl[][] [[0.0, 0.0, 0.0, 10.72, 3.0, 58.0], [1.0, 0.0, 0.0, 10.72, 3.0, 58.0], [2.0, 0.0, 0.0, 10.72, 3.0, 58.0], [3.0, 0.0, 0.0, 10.72, 3.0, 58.0], [4.0, 0.0, 0.0, 10.72, 3.0, 58.0], [5.0, 0.0, 0.0, 10.72, 3.0, 58.0]], "PreDraw Enum"=HEWH_PreDraw."" ("24 Hour PreDraw Enum")) -> (w58:T24)
            n36 = call <vilib>:"Add State(s) to Queue__jki_lib_state_machine.vi"("State(s) in Front (\"\")"="Read Dispense Time\nRead Remaining\nDisplay and Exit\nMacro: Exit", "State(s) in (\"\")"=w61) -> ("States Out"=w60:string)  [unwired: 13 in]
          }
          event Value Change {
            n37 = event-data() -> ("NewVal"=w67:T21)  [unwired: 1 in, 5 out]
            n38 = Bundle By Name(cluster=w69, "PreDraw Enum"=w67) -> (w68:T24)
            n39 = call <vilib>:"Add State(s) to Queue__jki_lib_state_machine.vi"("State(s) in Front (\"\")"="Check Tab" ("State(s) in Front (\"\")"), "State(s) in (\"\")"=w66) -> ("States Out"=w65:string)  [unwired: 13 in]
          }
          event "Low Usage": Value Change {
            n40 = event-data() -> ()  [unwired: 1 in, 6 out]
            n41 = Bundle By Name(cluster=w74, "Pattern Setup"=dbl[][] [[0.0, 0.0, 0.0, 15.0, 1.7, 58.0], [0.0, 30.0, 0.0, 2.0, 1.0, 58.0], [1.0, 0.0, 0.0, 1.0, 1.0, 58.0], [10.0, 30.0, 0.0, 6.0, 1.7, 58.0], [11.0, 30.0, 0.0, 4.0, 1.7, 58.0], [12.0, 0.0, 0.0, 1.0, 1.0, 58.0], [12.0, 45.0, 0.0, 1.0, 1.0, 58.0], [12.0, 50.0, 0.0, 1.0, 1.0, 58.0], [16.0, 15.0, 0.0, 2.0, 1.0, 58.0], [16.0, 45.0, 0.0, 2.0, 1.7, 58.0], [17.0, 0.0, 0.0, 3.0, 1.7, 58.0]], "PreDraw Enum"=HEWH_PreDraw."" ("24 Hour PreDraw Enum")) -> (w73:T24)
            n42 = call <vilib>:"Add State(s) to Queue__jki_lib_state_machine.vi"("State(s) in Front (\"\")"="Read Dispense Time\nRead Remaining\nDisplay and Exit\nMacro: Exit", "State(s) in (\"\")"=w77) -> ("States Out"=w76:string)  [unwired: 13 in]
          }
          event "Medium Usage": Value Change {
            n43 = event-data() -> ()  [unwired: 1 in, 6 out]
            n44 = Bundle By Name(cluster=w82, "Pattern Setup"=dbl[][] [[0.0, 0.0, 0.0, 15.0, 1.7, 58.0], [0.0, 30.0, 0.0, 2.0, 1.0, 58.0], [1.0, 40.0, 0.0, 9.0, 1.7, 58.0], [10.0, 30.0, 0.0, 9.0, 1.7, 58.0], [11.0, 30.0, 0.0, 5.0, 1.7, 58.0], [12.0, 0.0, 0.0, 1.0, 1.0, 58.0], [12.0, 45.0, 0.0, 1.0, 1.0, 58.0], [12.0, 50.0, 0.0, 1.0, 1.0, 58.0], [16.0, 0.0, 0.0, 1.0, 1.0, 58.0], [16.0, 15.0, 0.0, 2.0, 1.0, 58.0], [16.0, 45.0, 0.0, 2.0, 1.7, 58.0], [17.0, 0.0, 0.0, 7.0, 1.7, 58.0]], "PreDraw Enum"=HEWH_PreDraw."" ("24 Hour PreDraw Enum")) -> (w81:T24)
            n45 = call <vilib>:"Add State(s) to Queue__jki_lib_state_machine.vi"("State(s) in Front (\"\")"="Read Dispense Time\nRead Remaining\nDisplay and Exit\nMacro: Exit", "State(s) in (\"\")"=w85) -> ("States Out"=w84:string)  [unwired: 13 in]
          }
          event "High Usage": Value Change {
            n46 = event-data() -> ()  [unwired: 1 in, 6 out]
            n47 = Bundle By Name(cluster=w90, "Pattern Setup"=dbl[][] [[0.0, 0.0, 0.0, 27.0, 3.0, 58.0], [0.0, 30.0, 0.0, 2.0, 1.0, 58.0], [0.0, 40.0, 0.0, 1.0, 1.0, 58.0], [1.0, 40.0, 0.0, 9.0, 1.7, 58.0], [10.0, 30.0, 0.0, 15.0, 3.0, 58.0], [11.0, 30.0, 0.0, 5.0, 1.7, 58.0], [12.0, 0.0, 0.0, 1.0, 1.0, 58.0], [12.0, 45.0, 0.0, 1.0, 1.0, 58.0], [12.0, 50.0, 0.0, 1.0, 1.0, 58.0], [16.0, 0.0, 0.0, 2.0, 1.0, 58.0], [16.0, 15.0, 0.0, 2.0, 1.0, 58.0], [16.0, 30.0, 0.0, 2.0, 1.7, 58.0], [16.0, 45.0, 0.0, 2.0, 1.7, 58.0], [17.0, 0.0, 0.0, 14.0, 3.0, 58.0]], "PreDraw Enum"=HEWH_PreDraw."" ("24 Hour PreDraw Enum")) -> (w89:T24)
            n48 = call <vilib>:"Add State(s) to Queue__jki_lib_state_machine.vi"("State(s) in Front (\"\")"="Read Dispense Time\nRead Remaining\nDisplay and Exit\nMacro: Exit", "State(s) in (\"\")"=w93) -> ("States Out"=w92:string)  [unwired: 13 in]
          }
          event "Any Heat (1)": Value Change {
            n49 = event-data() -> ("NewVal"=w98:bool)  [unwired: 1 in, 5 out]
            n50 = Bundle By Name(cluster=w100, "Any Heat (1)"=w98) -> (w99:T24)
            n51 = call <vilib>:"Add State(s) to Queue__jki_lib_state_machine.vi"("State(s) in Front (\"\")"="Check for Draw Until" ("State(s) in Front (\"\")"), "State(s) in (\"\")"=w97) -> ("States Out"=w96:string)  [unwired: 13 in]
          }
          event "Any Heat (2)": Value Change {
            n52 = event-data() -> ("NewVal"=w102:bool)  [unwired: 1 in, 5 out]
            n53 = Bundle By Name(cluster=w104, "Any Heat (2)"=w102) -> (w103:T24)
            n54 = call <vilib>:"Add State(s) to Queue__jki_lib_state_machine.vi"("State(s) in Front (\"\")"="Check for Draw Until" ("State(s) in Front (\"\")"), "State(s) in (\"\")"=w107) -> ("States Out"=w106:string)  [unwired: 13 in]
          }
          event "Any Heat (3)": Value Change {
            n55 = event-data() -> ("NewVal"=w109:bool)  [unwired: 1 in, 5 out]
            n56 = Bundle By Name(cluster=w111, "Any Heat (3)"=w109) -> (w110:T24)
            n57 = call <vilib>:"Add State(s) to Queue__jki_lib_state_machine.vi"("State(s) in Front (\"\")"="Check for Draw Until" ("State(s) in Front (\"\")"), "State(s) in (\"\")"=w113) -> ("States Out"=w114:string)  [unwired: 13 in]
          }
          event Panel Close? {
            n58 = event-data() -> ()  [unwired: 1 in, 1 out]
            n59 = event-data("Discard?"=TRUE) -> ()  [unwired: 1 in, 1 out]
            n60 = call <vilib>:"Add State(s) to Queue__jki_lib_state_machine.vi"("State(s) in Front (\"\")"="Macro: Exit", "State(s) in (\"\")"=w121) -> ("States Out"=w120:string)  [unwired: 13 in]
          }
          event "Draw Pattern Setup Tab": Value Change {
            n61 = event-data() -> ()  [unwired: 1 in, 6 out]
            n62 = local read "Draw Pattern Setup Tab"() -> (w124:T20)
            n63 = local read "Draw Pattern Setup Tab"() -> (w123:T20)
            n64 = Equal?(x=w124, y=T20."Standard Pattern" ("Draw Pattern Setup")) -> (x = y?=w126:bool)
            n65 = Equal?(x=w123, y=T20."Pre-Draw Setup" ("Draw Pattern Setup")) -> (x = y?=w127:bool)
            n66 = case shown="False" w127 {
              frame False {
                n67 = property on="24 Hour PreDraw Enum" class="Enum (strict)"("Visible"=FALSE) -> ()  [unwired: 2 in, 2 out]
              }
              frame True {
                n68 = property on="24 Hour PreDraw Enum" class="Enum (strict)"("Visible"=TRUE) -> ()  [unwired: 2 in, 2 out]
              }
            }
            n69 = case shown="True" w126 {
              frame False {
                n70 = property on="stop" class="Bool"("Visible"=TRUE) -> ()  [unwired: 2 in, 2 out]
              }
              frame True {
                n71 = property on="stop" class="Bool"("Visible"=FALSE) -> ()  [unwired: 2 in, 2 out]
              }
            }
          }
          event "Populate High Usage": Value Change {
            w136 = dbl[][] [[0.0, 0.0, 0.0, 27.0, 3.0, 58.0], [0.0, 30.0, 0.0, 2.0, 1.0, 58.0], [0.0, 40.0, 0.0, 1.0, 1.0, 58.0], [1.0, 40.0, 0.0, 9.0, 1.7, 58.0], [10.0, 30.0, 0.0, 15.0, 3.0, 58.0], [11.0, 30.0, 0.0, 5.0, 1.7, 58.0], [12.0, 0.0, 0.0, 1.0, 1.0, 58.0], [12.0, 45.0, 0.0, 1.0, 1.0, 58.0], [12.0, 50.0, 0.0, 1.0, 1.0, 58.0], [16.0, 0.0, 0.0, 2.0, 1.0, 58.0], [16.0, 15.0, 0.0, 2.0, 1.0, 58.0], [16.0, 30.0, 0.0, 2.0, 1.7, 58.0], [16.0, 45.0, 0.0, 2.0, 1.7, 58.0], [17.0, 0.0, 0.0, 14.0, 3.0, 58.0]]  # High Usage
            n72 = event-data() -> ()  [unwired: 1 in, 6 out]
            n73 = Bundle By Name(cluster=w138, "Pattern Setup"=w136) -> (w137:T24)
            n74 = local write "Pattern Setup"(w136) -> ()
          }
          event "Populate Medium Usage": Value Change {
            w141 = dbl[][] [[0.0, 0.0, 0.0, 15.0, 1.7, 58.0], [0.0, 30.0, 0.0, 2.0, 1.0, 58.0], [1.0, 40.0, 0.0, 9.0, 1.7, 58.0], [10.0, 30.0, 0.0, 9.0, 1.7, 58.0], [11.0, 30.0, 0.0, 5.0, 1.7, 58.0], [12.0, 0.0, 0.0, 1.0, 1.0, 58.0], [12.0, 45.0, 0.0, 1.0, 1.0, 58.0], [12.0, 50.0, 0.0, 1.0, 1.0, 58.0], [16.0, 0.0, 0.0, 1.0, 1.0, 58.0], [16.0, 15.0, 0.0, 2.0, 1.0, 58.0], [16.0, 45.0, 0.0, 2.0, 1.7, 58.0], [17.0, 0.0, 0.0, 7.0, 1.7, 58.0]]  # Medium Usage
            n75 = event-data() -> ()  [unwired: 1 in, 6 out]
            n76 = local write "Pattern Setup"(w141) -> ()
            n77 = Bundle By Name(cluster=w143, "Pattern Setup"=w141) -> (w142:T24)
          }
          event "Populate Low Usage": Value Change {
            w146 = dbl[][] [[0.0, 0.0, 0.0, 15.0, 1.7, 58.0], [0.0, 30.0, 0.0, 2.0, 1.0, 58.0], [1.0, 0.0, 0.0, 1.0, 1.0, 58.0], [10.0, 30.0, 0.0, 6.0, 1.7, 58.0], [11.0, 30.0, 0.0, 4.0, 1.7, 58.0], [12.0, 0.0, 0.0, 1.0, 1.0, 58.0], [12.0, 45.0, 0.0, 1.0, 1.0, 58.0], [12.0, 50.0, 0.0, 1.0, 1.0, 58.0], [16.0, 15.0, 0.0, 2.0, 1.0, 58.0], [16.0, 45.0, 0.0, 2.0, 1.7, 58.0], [17.0, 0.0, 0.0, 3.0, 1.7, 58.0]]  # Low Usage
            n78 = event-data() -> ()  [unwired: 1 in, 6 out]
            n79 = Bundle By Name(cluster=w148, "Pattern Setup"=w146) -> (w147:T24)
            n80 = local write "Pattern Setup"(w146) -> ()
          }
          event "Populate Older": Value Change {
            w150 = dbl[][] [[0.0, 0.0, 0.0, 10.72, 3.0, 58.0], [1.0, 0.0, 0.0, 10.72, 3.0, 58.0], [2.0, 0.0, 0.0, 10.72, 3.0, 58.0], [3.0, 0.0, 0.0, 10.72, 3.0, 58.0], [4.0, 0.0, 0.0, 10.72, 3.0, 58.0], [5.0, 0.0, 0.0, 10.72, 3.0, 58.0]]  # Older
            n81 = event-data() -> ()  [unwired: 1 in, 6 out]
            n82 = local write "Pattern Setup"(w150) -> ()
            n83 = Bundle By Name(cluster=w153, "Pattern Setup"=w150) -> (w152:T24)
          }
        }
      }
      frame "---------- Core ----------" {
        # "Do not put any code in this frame.\n(it is a separator no-op)"
        n84 = call <vilib>:"Add State(s) to Queue__jki_lib_state_machine.vi"("State(s) in (\"\")"=w158) -> ("States Out"=w157:string)  [unwired: 14 in]
      }
      frame Default {
        w168 = 42 items=["No error", "Argument error", "Memory is full", "Out of zone", "End of file", "File already open", "Generic file I/O error", "File not found", "File permission error", "Disk is full", "Duplicate path", "Too many files open", "System feature not enabled", "Resource file not found", "Cannot add resource", "Resource not found", "Image not found", "Image memory error", "Pen does not exist", "Config type invalid", "Config token not found", "Config parse error", "Config memory error", "Bad external code format", "Bad external code offset", "External code not present", "Null window", "Destroy window error", "Null menu", "Print aborted", "Bad print record", "Print driver error", "Windows error during printing", "Memory error during printing", "Print dialog error", "Generic print error", "Invalid device refnum", "Device not found", "Device parameter error", "Device unit error", "Cannot open device", "Device call aborted", "Generic error", "Cancelled by user", "Object ID too low", "Object ID too high", "Object not in heap", "Unknown heap", "Unknown object (invalid DefProc)", "Unknown object (DefProc not in table)", "Message out of range", "Invalid (null) method", "Unknown message", "Manager call not supported", "Bad address", "Network operation in progress", "Network operation timed out", "Connection is busy", "Network attribute not supported", "Network error", "Address in use", "System out of memory", "Connection aborted", "Connection refused", "Not connected", "Already connected", "Connection closed", "Initialization error (interapplication manager)", "Bad occurrence", "Wait on unbound occurrence handler", "Occurrence queue overflow", "Datalog type conflict", "Unused", "Unrecognized type (interapplication manager)", "Memory corrupt", "Failed to make temporary DLL", "Old CIN version", "Drag socket not found", "Failed to load drop-object", "Failed to register OLE object", "Failed to release OLE object", "Format specifier type mismatch", "Unknown format specifier", "Too few format specifiers", "Too many format specifiers", "Scan failed", "Newer CIN version", "Error converting to variant", "Runtime menu error", "Password tampered", "Variant attribute not found", "Incompatible variant data type", "Event data is not available", "Event Store is not present", "Occurrence is not found", "Event Queue is not created", "Event info is not available", "Refnum passed is NULL", "Error retrieving Class GUID", "Error retrieving CoClass GUID", "Error retrieving TypeLib GUID.", "Bad built application magic bytes.", "Specific driver is different from the specific driver associated with the Logical Name.", "There is no session opened to the class driver.", "Max Error", "MAX - Error with config objects", "MAX - Error loading configuration", "MAX - Group not supported"]
        # "Current State"
        # "Do not delete, rename, or modify this frame.\n(this is used to capture unhandled states and typos)"
        # "Handle mistyped state name (developer tool)"
        n85 = Format Into String(format string="Software Exception: Unhandled State \"%s\"." ("message"), error in=w164, w159) -> (resulting string=w167:string, error out=w166:errorcluster)  [unwired: 1 in]
        n86 = call <vilib>:"Error Cluster From Error Code.vi"("show call chain? (False)"=TRUE, "error in (no error)"=w166, "error message (\"\")"=w167, "error code (0)"=w168) -> ("error out"=w165:errorcluster)  [unwired: 5 in]
        n87 = call <vilib>:"Add State(s) to Queue__jki_lib_state_machine.vi"("State(s) in (\"\")"=w163) -> ("States Out"=w162:string)  [unwired: 14 in]
      }
      frame "Initialize Core Data" {
        # "Do not delete, rename, or modify this frame.\n(this is used to determine panel behavior on exit)"
        # "originally closed?"
        # "exe?"
        # "If panel starts closed or is an EXE, then close it when we exit"
        n88 = property class="VI"() -> ("Front Panel.Open"=w177:bool)  [unwired: 2 in, 2 out]
        n89 = property class="App"() -> ("App.Kind"=w176:T22)  [unwired: 2 in, 2 out]
        n90 = control-ref of="Current VI Reference"() -> (w170:refnum<vi>)
        n91 = Not(x=w177) -> (.not. x?=w174:bool)
        n92 = Equal?(x=w176, y=T22."Run Time System" ("Application:Kind")) -> (x = y?=w173:bool)
        n93 = Or(x=w174, y=w173) -> (x .or. y?=w171:bool)
        n94 = Bundle By Name(cluster=w172, "Core.Current VI Reference"=w170, "Core.Close Panel on Exit?"=w171) -> (w179:T24)
        n95 = call <vilib>:"Add State(s) to Queue__jki_lib_state_machine.vi"("State(s) in (\"\")"=w181) -> ("States Out"=w180:string)  [unwired: 14 in]
      }
      frame "Error Handler" {
        # "Unhandled Error -- Display it"
        # "Handle any errors here.\nYou can also output any states to clean-up after errors occur"
        # "Clear error"
        n96 = call <vilib>:"General Error Handler.vi"("error in (no error)"=w183) -> ()  [unwired: 10 in, 5 out]
        n97 = call <vilib>:"Add State(s) to Queue__jki_lib_state_machine.vi"("State(s) in Front (\"\")"="/* Post Error States", "State(s) in (\"\")"=w187) -> ("States Out"=w186:string)  [unwired: 13 in]
      }
      frame "Exit" {
        # "Do not put any code in this frame.\n(No errors that occur here will be handled.)"
        n98 = call <vilib>:"Add State(s) to Queue__jki_lib_state_machine.vi"("State(s) in (\"\")"=w192) -> ("States Out"=w191:string)  [unwired: 14 in]
      }
      frame "---------- Data ----------" {
        # "Do not put any code in this frame.\n(It is a separator no-op. You can make a copy of this frame to create a new Data frame)"
        n99 = call <vilib>:"Add State(s) to Queue__jki_lib_state_machine.vi"("State(s) in (\"\")"=w196) -> ("States Out"=w195:string)  [unwired: 14 in]
      }
      frame "Data: Initialize" {
        w203 = T25 {"Current VI Reference"=refnum, "Close Panel on Exit?"=FALSE}  # Core
        n100 = Bundle("Core"=w203, "Pattern Setup"="Pattern Setup", "Core HEWH Data Input"="Core HEWH Data Input", "PreDraw Enum"="PreDraw Enum", "Any Heat (1)"="Any Heat (1)", "Any Heat (2)"="Any Heat (2)", "Any Heat (3)"="Any Heat (3)") -> (w205:T24)  [unwired: 1 in]
        n101 = call <vilib>:"Add State(s) to Queue__jki_lib_state_machine.vi"("State(s) in (\"\")"=w207) -> ("States Out"=w206:string)  [unwired: 14 in]
      }
      frame "Data: Cleanup" {
        # "Cleanup any data and references, here.\n(this is called automatically, by the Macro: Exit)"
        n102 = Unbundle By Name(w208) -> ("Core.Current VI Reference"=w211:refnum<vi>)
        n103 = Close Reference(reference=w211, error in (no error)=w210) -> (error out=w209:errorcluster)
        n104 = call <vilib>:"Add State(s) to Queue__jki_lib_state_machine.vi"("State(s) in (\"\")"=w213) -> ("States Out"=w212:string)  [unwired: 14 in]
      }
      frame "---------- UI ----------" {
        # "Do not put any code in this frame.\n(It is a separator no-op. You can make a copy of this frame to create a new UI frame)"
        n105 = call <vilib>:"Add State(s) to Queue__jki_lib_state_machine.vi"("State(s) in (\"\")"=w217) -> ("States Out"=w216:string)  [unwired: 14 in]
      }
      frame "UI: Initialize" {
        w219 = FALSE ("Visible")
        w218 = FALSE ("Visible")
        w220 = FALSE ("Visible")
        w221 = FALSE ("Visible")
        w222 = FALSE ("Visible")
        # "Initialize the User Interface, here.\n(this is called automatically, by the Macro: Init)"
        n106 = property on="Description 4" class="Str"("Visible"=w219) -> ()  [unwired: 2 in, 2 out]
        n107 = property on="Description 5" class="Str"("Visible"=w219) -> ()  [unwired: 2 in, 2 out]
        n108 = property on="Description 6" class="Str"("Visible"=w219) -> ()  [unwired: 2 in, 2 out]
        n109 = property on="Description 1" class="Str"("Visible"=w222) -> ()  [unwired: 2 in, 2 out]
        n110 = property on="Total Gallons (1)" class="DigNum (strict)"("Visible"=w222) -> ()  [unwired: 2 in, 2 out]
        n111 = property on="Flow Rate (GPM 1)" class="DigNum (strict)"("Visible"=w222) -> ()  [unwired: 2 in, 2 out]
        n112 = property on="Incoming Water Temperature (1)" class="DigNum (strict)"("Visible"=w222) -> ()  [unwired: 2 in, 2 out]
        n113 = property on="Incoming Water Temperature (2)" class="DigNum (strict)"("Visible"=w220) -> ()  [unwired: 2 in, 2 out]
        n114 = property on="Description 2" class="Str"("Visible"=w220) -> ()  [unwired: 2 in, 2 out]
        n115 = property on="Total Gallons (2)" class="DigNum (strict)"("Visible"=w220) -> ()  [unwired: 2 in, 2 out]
        n116 = property on="Flow Rate (GPM 2)" class="DigNum (strict)"("Visible"=w220) -> ()  [unwired: 2 in, 2 out]
        n117 = property on="Description 3" class="Str"("Visible"=w221) -> ()  [unwired: 2 in, 2 out]
        n118 = property on="Total Gallons (3)" class="DigNum (strict)"("Visible"=w221) -> ()  [unwired: 2 in, 2 out]
        n119 = property on="Flow Rate (GPM 3)" class="DigNum (strict)"("Visible"=w221) -> ()  [unwired: 2 in, 2 out]
        n120 = property on="Incoming Water Temperature (3)" class="DigNum (strict)"("Visible"=w221) -> ()  [unwired: 2 in, 2 out]
        n121 = property on="Any Heat (1)" class="Bool (strict)"("Visible"=w218) -> ()  [unwired: 2 in, 2 out]
        n122 = property on="Any Heat (2)" class="Bool (strict)"("Visible"=w218) -> ()  [unwired: 2 in, 2 out]
        n123 = property on="Any Heat (3)" class="Bool (strict)"("Visible"=w218) -> ()  [unwired: 2 in, 2 out]
        n124 = call <vilib>:"Add State(s) to Queue__jki_lib_state_machine.vi"("State(s) in (\"\")"=w226) -> ("States Out"=w225:string)  [unwired: 14 in]
      }
      frame "UI: Cursor Set" {
        # "Argument"
        # "Set and Unset Cursor Busy.\n(Usage: \"UI: Cursor Set >> Busy|Idle\")"
        n125 = case shown="\"Idle\", Default" w227 {
          tunnel: w229 -> [w234 w236]
          tunnel: [w233 w235] -> w228
          frame "Idle", Default {
            n126 = call <vilib>:"Unset Busy.vi"("error in (no error)"=w234) -> ("error out"=w233:errorcluster)  [unwired: 10 in]
          }
          frame "Busy" {
            n127 = call <vilib>:"Set Busy.vi"("error in (no error)"=w236) -> ("error out"=w235:errorcluster)  [unwired: 9 in, 1 out]
          }
        }
        n128 = call <vilib>:"Add State(s) to Queue__jki_lib_state_machine.vi"("State(s) in (\"\")"=w232) -> ("States Out"=w231:string)  [unwired: 14 in]
      }
      frame "UI: Front Panel State" {
        # "Argument"
        # "Set Front Panel Open or Closed\n(Usage: \"UI: Front Panel State >> Open|Close\")"
        n129 = Unbundle By Name(w239) -> ("Core.Current VI Reference"=w238:refnum<vi>)
        n130 = case shown="\"Open\", Default" w237 {
          tunnel: w241 -> [w247 w260]
          tunnel: [w249 w261] -> w240
          tunnel: w238 -> [w248 w258]
          frame "Open", Default {
            n131 = property class="VI"(reference=w248, error in=w247) -> (reference out=w245:refnum<vi>, error out=w246:errorcluster, "Front Panel.Open"=w244:bool)
            n132 = case shown="False" w244 {
              tunnel: [w252 w255] -> w249
              tunnel: w246 -> [w251 w255]
              tunnel: w245 -> [w250 _]
              frame False {
                n133 = invoke class="VI" method="FP.Open"(reference=w250, error in=w251, "Activate"=TRUE, "State"=T23."Standard") -> (error out=w252:errorcluster)  [unwired: 1 in, 4 out]
              }
              frame True {
              }
            }
          }
          frame "Close" {
            n134 = property class="VI"(reference=w258, error in=w260) -> (reference out=w257:refnum<vi>, error out=w259:errorcluster, "Front Panel.Open"=w256:bool)
            n135 = case shown="True" w256 {
              tunnel: [w262 w265] -> w261
              tunnel: w259 -> [w262 w264]
              tunnel: w257 -> [_ w263]
              frame False {
              }
              frame True {
                n136 = invoke class="VI" method="FP.Close"(reference=w263, error in=w264) -> (error out=w265:errorcluster)  [unwired: 1 in, 2 out]
              }
            }
          }
        }
        n137 = call <vilib>:"Add State(s) to Queue__jki_lib_state_machine.vi"("State(s) in (\"\")"=w243) -> ("States Out"=w242:string)  [unwired: 14 in]
      }
      frame "---------- Macro ----------" {
        # "Do not put any code in this frame.\n(It is a separator no-op. You can make a copy of this frame to create a new Macro frame)"
        n138 = call <vilib>:"Add State(s) to Queue__jki_lib_state_machine.vi"("State(s) in (\"\")"=w269) -> ("States Out"=w268:string)  [unwired: 14 in]
      }
      frame "Macro: Initialize" {
        w271 = "Data: Initialize\nInitialize Core Data\nUI: Initialize\nUI: Front Panel State >> Open"  # Data: Initialize Initialize Core Data UI: Initialize UI: Front Panel State >> Open
        n139 = call <vilib>:"Add State(s) to Queue__jki_lib_state_machine.vi"("State(s) in Front (\"\")"=w271, "State(s) in (\"\")"=w274) -> ("States Out"=w273:string)  [unwired: 13 in]
      }
      frame "Macro: Exit" {
        # "Exit Macro\n(This is called once, when the VI exits)"
        n140 = Unbundle By Name(w281) -> ("Core.Close Panel on Exit?"=w280:bool)
        n141 = Select(t="UI: Front Panel State >> Close", s=w280, f="") -> (s? t:f=w277:string)
        n142 = call <vilib>:"Add State(s) to Queue__jki_lib_state_machine.vi"("State(s) in (\"\")"=w277, "State(s) at Back (\"\")"="Data: Cleanup\nExit") -> ("States Out"=w275:string)  [unwired: 13 in]
        n143 = call <vilib>:"Add State(s) to Queue__jki_lib_state_machine.vi"("State(s) in Front (\"\")"=w275, "State(s) in (\"\")"=w284) -> ("States Out"=w283:string)  [unwired: 13 in]
      }
      frame "---------- New Category ----------" {
        # "Template Separator\n(You can make a copy of, or modify, this frame)"
        n144 = call <vilib>:"Add State(s) to Queue__jki_lib_state_machine.vi"("State(s) in (\"\")"=w288) -> ("States Out"=w287:string)  [unwired: 14 in]
      }
      frame "Check Tab" {
        n145 = Unbundle By Name(w290) -> ("PreDraw Enum"=w289:T21)
        n146 = case shown="\"Zero Pre-Draws\", Default" w289 {
          frame "Zero Pre-Draws", Default {
            w294 = FALSE ("Visible")
            w295 = FALSE ("Visible")
            w296 = FALSE ("Visible")
            w297 = FALSE ("Visible")
            w298 = FALSE ("Visible")
            n147 = property on="Description 1" class="Str"("Visible"=w298) -> ()  [unwired: 2 in, 2 out]
            n148 = property on="Total Gallons (1)" class="DigNum (strict)"("Visible"=w298) -> ()  [unwired: 2 in, 2 out]
            n149 = property on="Flow Rate (GPM 1)" class="DigNum (strict)"("Visible"=w298) -> ()  [unwired: 2 in, 2 out]
            n150 = property on="Incoming Water Temperature (1)" class="DigNum (strict)"("Visible"=w298) -> ()  [unwired: 2 in, 2 out]
            n151 = property on="Incoming Water Temperature (2)" class="DigNum (strict)"("Visible"=w296) -> ()  [unwired: 2 in, 2 out]
            n152 = property on="Description 2" class="Str"("Visible"=w296) -> ()  [unwired: 2 in, 2 out]
            n153 = property on="Total Gallons (2)" class="DigNum (strict)"("Visible"=w296) -> ()  [unwired: 2 in, 2 out]
            n154 = property on="Flow Rate (GPM 2)" class="DigNum (strict)"("Visible"=w296) -> ()  [unwired: 2 in, 2 out]
            n155 = property on="Description 3" class="Str"("Visible"=w297) -> ()  [unwired: 2 in, 2 out]
            n156 = property on="Total Gallons (3)" class="DigNum (strict)"("Visible"=w297) -> ()  [unwired: 2 in, 2 out]
            n157 = property on="Flow Rate (GPM 3)" class="DigNum (strict)"("Visible"=w297) -> ()  [unwired: 2 in, 2 out]
            n158 = property on="Incoming Water Temperature (3)" class="DigNum (strict)"("Visible"=w297) -> ()  [unwired: 2 in, 2 out]
            n159 = property on="Description 4" class="Str"("Visible"=w295) -> ()  [unwired: 2 in, 2 out]
            n160 = property on="Description 5" class="Str"("Visible"=w295) -> ()  [unwired: 2 in, 2 out]
            n161 = property on="Description 6" class="Str"("Visible"=w295) -> ()  [unwired: 2 in, 2 out]
            n162 = property on="Any Heat (1)" class="Bool (strict)"("Visible"=w294) -> ()  [unwired: 2 in, 2 out]
            n163 = property on="Any Heat (2)" class="Bool (strict)"("Visible"=w294) -> ()  [unwired: 2 in, 2 out]
            n164 = property on="Any Heat (3)" class="Bool (strict)"("Visible"=w294) -> ()  [unwired: 2 in, 2 out]
          }
          frame "One Pre- Draws" {
            w299 = FALSE ("Visible")
            w301 = FALSE ("Visible")
            w303 = FALSE ("Visible")
            w304 = FALSE ("Visible")
            w305 = TRUE ("Visible")
            n165 = property on="Description 1" class="Str"("Visible"=w305) -> ()  [unwired: 2 in, 2 out]
            n166 = property on="Total Gallons (1)" class="DigNum (strict)"("Visible"=w305) -> ()  [unwired: 2 in, 2 out]
            n167 = property on="Flow Rate (GPM 1)" class="DigNum (strict)"("Visible"=w305) -> ()  [unwired: 2 in, 2 out]
            n168 = property on="Incoming Water Temperature (1)" class="DigNum (strict)"("Visible"=w305) -> ()  [unwired: 2 in, 2 out]
            n169 = property on="Description 2" class="Str"("Visible"=w303) -> ()  [unwired: 2 in, 2 out]
            n170 = property on="Total Gallons (2)" class="DigNum (strict)"("Visible"=w303) -> ()  [unwired: 2 in, 2 out]
            n171 = property on="Flow Rate (GPM 2)" class="DigNum (strict)"("Visible"=w303) -> ()  [unwired: 2 in, 2 out]
            n172 = property on="Incoming Water Temperature (2)" class="DigNum (strict)"("Visible"=w303) -> ()  [unwired: 2 in, 2 out]
            n173 = property on="Description 3" class="Str"("Visible"=w304) -> ()  [unwired: 2 in, 2 out]
            n174 = property on="Total Gallons (3)" class="DigNum (strict)"("Visible"=w304) -> ()  [unwired: 2 in, 2 out]
            n175 = property on="Flow Rate (GPM 3)" class="DigNum (strict)"("Visible"=w304) -> ()  [unwired: 2 in, 2 out]
            n176 = property on="Incoming Water Temperature (3)" class="DigNum (strict)"("Visible"=w304) -> ()  [unwired: 2 in, 2 out]
            n177 = property on="Description 4" class="Str"("Visible"=TRUE) -> ()  [unwired: 2 in, 2 out]
            n178 = property on="Description 5" class="Str"("Visible"=w301) -> ()  [unwired: 2 in, 2 out]
            n179 = property on="Description 6" class="Str"("Visible"=w301) -> ()  [unwired: 2 in, 2 out]
            n180 = property on="Any Heat (1)" class="Bool (strict)"("Visible"=TRUE) -> ()  [unwired: 2 in, 2 out]
            n181 = property on="Any Heat (2)" class="Bool (strict)"("Visible"=w299) -> ()  [unwired: 2 in, 2 out]
            n182 = property on="Any Heat (3)" class="Bool (strict)"("Visible"=w299) -> ()  [unwired: 2 in, 2 out]
          }
          frame "Two Pre-Draws" {
            w312 = TRUE ("Visible")
            w313 = FALSE ("Visible")
            w314 = TRUE ("Visible")
            n183 = property on="Description 1" class="Str"("Visible"=w314) -> ()  [unwired: 2 in, 2 out]
            n184 = property on="Total Gallons (1)" class="DigNum (strict)"("Visible"=w314) -> ()  [unwired: 2 in, 2 out]
            n185 = property on="Flow Rate (GPM 1)" class="DigNum (strict)"("Visible"=w314) -> ()  [unwired: 2 in, 2 out]
            n186 = property on="Incoming Water Temperature (1)" class="DigNum (strict)"("Visible"=w314) -> ()  [unwired: 2 in, 2 out]
            n187 = property on="Description 2" class="Str"("Visible"=w312) -> ()  [unwired: 2 in, 2 out]
            n188 = property on="Total Gallons (2)" class="DigNum (strict)"("Visible"=w312) -> ()  [unwired: 2 in, 2 out]
            n189 = property on="Flow Rate (GPM 2)" class="DigNum (strict)"("Visible"=w312) -> ()  [unwired: 2 in, 2 out]
            n190 = property on="Incoming Water Temperature (2)" class="DigNum (strict)"("Visible"=w312) -> ()  [unwired: 2 in, 2 out]
            n191 = property on="Description 3" class="Str"("Visible"=w313) -> ()  [unwired: 2 in, 2 out]
            n192 = property on="Total Gallons (3)" class="DigNum (strict)"("Visible"=w313) -> ()  [unwired: 2 in, 2 out]
            n193 = property on="Flow Rate (GPM 3)" class="DigNum (strict)"("Visible"=w313) -> ()  [unwired: 2 in, 2 out]
            n194 = property on="Incoming Water Temperature (3)" class="DigNum (strict)"("Visible"=w313) -> ()  [unwired: 2 in, 2 out]
            n195 = property on="Description 4" class="Str"("Visible"=TRUE) -> ()  [unwired: 2 in, 2 out]
            n196 = property on="Description 5" class="Str"("Visible"=TRUE) -> ()  [unwired: 2 in, 2 out]
            n197 = property on="Description 6" class="Str"("Visible"=FALSE) -> ()  [unwired: 2 in, 2 out]
            n198 = property on="Any Heat (1)" class="Bool (strict)"("Visible"=TRUE) -> ()  [unwired: 2 in, 2 out]
            n199 = property on="Any Heat (2)" class="Bool (strict)"("Visible"=TRUE) -> ()  [unwired: 2 in, 2 out]
            n200 = property on="Any Heat (3)" class="Bool (strict)"("Visible"=FALSE ("Any Heat (3)")) -> ()  [unwired: 2 in, 2 out]
          }
          frame "Three Pre-Draws" {
            w321 = TRUE ("Visible")
            w322 = TRUE ("Visible")
            w323 = TRUE ("Visible")
            n201 = property on="Description 1" class="Str"("Visible"=w323) -> ()  [unwired: 2 in, 2 out]
            n202 = property on="Total Gallons (1)" class="DigNum (strict)"("Visible"=w323) -> ()  [unwired: 2 in, 2 out]
            n203 = property on="Flow Rate (GPM 1)" class="DigNum (strict)"("Visible"=w323) -> ()  [unwired: 2 in, 2 out]
            n204 = property on="Incoming Water Temperature (1)" class="DigNum (strict)"("Visible"=w323) -> ()  [unwired: 2 in, 2 out]
            n205 = property on="Description 2" class="Str"("Visible"=w321) -> ()  [unwired: 2 in, 2 out]
            n206 = property on="Total Gallons (2)" class="DigNum (strict)"("Visible"=w321) -> ()  [unwired: 2 in, 2 out]
            n207 = property on="Flow Rate (GPM 2)" class="DigNum (strict)"("Visible"=w321) -> ()  [unwired: 2 in, 2 out]
            n208 = property on="Incoming Water Temperature (2)" class="DigNum (strict)"("Visible"=w321) -> ()  [unwired: 2 in, 2 out]
            n209 = property on="Description 3" class="Str"("Visible"=w322) -> ()  [unwired: 2 in, 2 out]
            n210 = property on="Total Gallons (3)" class="DigNum (strict)"("Visible"=w322) -> ()  [unwired: 2 in, 2 out]
            n211 = property on="Flow Rate (GPM 3)" class="DigNum (strict)"("Visible"=w322) -> ()  [unwired: 2 in, 2 out]
            n212 = property on="Incoming Water Temperature (3)" class="DigNum (strict)"("Visible"=w322) -> ()  [unwired: 2 in, 2 out]
            n213 = property on="Any Heat (2)" class="Bool (strict)"("Visible"=TRUE) -> ()  [unwired: 2 in, 2 out]
            n214 = property on="Any Heat (1)" class="Bool (strict)"("Visible"=TRUE) -> ()  [unwired: 2 in, 2 out]
            n215 = property on="Any Heat (3)" class="Bool (strict)"("Visible"=TRUE ("Any Heat (3)")) -> ()  [unwired: 2 in, 2 out]
            n216 = property on="Description 4" class="Str"("Visible"=TRUE) -> ()  [unwired: 2 in, 2 out]
            n217 = property on="Description 5" class="Str"("Visible"=TRUE) -> ()  [unwired: 2 in, 2 out]
            n218 = property on="Description 6" class="Str"("Visible"=TRUE) -> ()  [unwired: 2 in, 2 out]
          }
        }
        n219 = call <vilib>:"Add State(s) to Queue__jki_lib_state_machine.vi"("State(s) in (\"\")"=w293) -> ("States Out"=w292:string)  [unwired: 14 in]
      }
      frame "Check for Draw Until" {
        n220 = Unbundle By Name(w328) -> ("PreDraw Enum"=w327:T21, "Any Heat (1)"=w326:bool, "Any Heat (2)"=w325:bool, "Any Heat (3)"=w324:bool)
        n221 = case shown="\"One Pre- Draws\"" w327 {
          tunnel: w326 -> [_ w339 w342 w350]
          tunnel: w325 -> [_ _ w344 w349]
          tunnel: w324 -> [_ _ _ w351]
          frame "Zero Pre-Draws", Default {
            w332 = FALSE ("Visible")
            w333 = FALSE ("Visible")
            w334 = FALSE ("Visible")
            w335 = FALSE ("Visible")
            w336 = FALSE ("Visible")
            n222 = property on="Description 1" class="Str"("Visible"=w336) -> ()  [unwired: 2 in, 2 out]
            n223 = property on="Total Gallons (1)" class="DigNum (strict)"("Visible"=w336) -> ()  [unwired: 2 in, 2 out]
            n224 = property on="Flow Rate (GPM 1)" class="DigNum (strict)"("Visible"=w336) -> ()  [unwired: 2 in, 2 out]
            n225 = property on="Incoming Water Temperature (1)" class="DigNum (strict)"("Visible"=w336) -> ()  [unwired: 2 in, 2 out]
            n226 = property on="Incoming Water Temperature (2)" class="DigNum (strict)"("Visible"=w335) -> ()  [unwired: 2 in, 2 out]
            n227 = property on="Description 2" class="Str"("Visible"=w335) -> ()  [unwired: 2 in, 2 out]
            n228 = property on="Total Gallons (2)" class="DigNum (strict)"("Visible"=w335) -> ()  [unwired: 2 in, 2 out]
            n229 = property on="Flow Rate (GPM 2)" class="DigNum (strict)"("Visible"=w335) -> ()  [unwired: 2 in, 2 out]
            n230 = property on="Description 3" class="Str"("Visible"=w334) -> ()  [unwired: 2 in, 2 out]
            n231 = property on="Total Gallons (3)" class="DigNum (strict)"("Visible"=w334) -> ()  [unwired: 2 in, 2 out]
            n232 = property on="Flow Rate (GPM 3)" class="DigNum (strict)"("Visible"=w334) -> ()  [unwired: 2 in, 2 out]
            n233 = property on="Incoming Water Temperature (3)" class="DigNum (strict)"("Visible"=w334) -> ()  [unwired: 2 in, 2 out]
            n234 = property on="Description 4" class="Str"("Visible"=w333) -> ()  [unwired: 2 in, 2 out]
            n235 = property on="Description 5" class="Str"("Visible"=w333) -> ()  [unwired: 2 in, 2 out]
            n236 = property on="Description 6" class="Str"("Visible"=w333) -> ()  [unwired: 2 in, 2 out]
            n237 = property on="Any Heat (1)" class="Bool (strict)"("Visible"=w332) -> ()  [unwired: 2 in, 2 out]
            n238 = property on="Any Heat (2)" class="Bool (strict)"("Visible"=w332) -> ()  [unwired: 2 in, 2 out]
            n239 = property on="Any Heat (3)" class="Bool (strict)"("Visible"=w332) -> ()  [unwired: 2 in, 2 out]
          }
          frame "One Pre- Draws" {
            w337 = FALSE ("Visible")
            w338 = FALSE ("Visible")
            n240 = case shown="True" w339 {
              frame False {
                w340 = TRUE ("Visible")
                n241 = property on="Description 1" class="Str"("Visible"=w340) -> ()  [unwired: 2 in, 2 out]
                n242 = property on="Total Gallons (1)" class="DigNum (strict)"("Visible"=w340) -> ()  [unwired: 2 in, 2 out]
                n243 = property on="Incoming Water Temperature (1)" class="DigNum (strict)"("Visible"=w340) -> ()  [unwired: 2 in, 2 out]
                n244 = property on="Flow Rate (GPM 1)" class="DigNum (strict)"("Visible"=w340) -> ()  [unwired: 2 in, 2 out]
              }
              frame True {
                w341 = FALSE ("Visible")
                n245 = property on="Description 1" class="Str"("Visible"=w341) -> ()  [unwired: 2 in, 2 out]
                n246 = property on="Total Gallons (1)" class="DigNum (strict)"("Visible"=w341) -> ()  [unwired: 2 in, 2 out]
                n247 = property on="Incoming Water Temperature (1)" class="DigNum (strict)"("Visible"=w341) -> ()  [unwired: 2 in, 2 out]
                n248 = property on="Flow Rate (GPM 1)" class="DigNum (strict)"("Visible"=w341) -> ()  [unwired: 2 in, 2 out]
              }
            }
            n249 = property on="Description 3" class="Str"("Visible"=w337) -> ()  [unwired: 2 in, 2 out]
            n250 = property on="Description 2" class="Str"("Visible"=w338) -> ()  [unwired: 2 in, 2 out]
            n251 = property on="Total Gallons (3)" class="DigNum (strict)"("Visible"=w337) -> ()  [unwired: 2 in, 2 out]
            n252 = property on="Total Gallons (2)" class="DigNum (strict)"("Visible"=w338) -> ()  [unwired: 2 in, 2 out]
            n253 = property on="Incoming Water Temperature (3)" class="DigNum (strict)"("Visible"=w337) -> ()  [unwired: 2 in, 2 out]
            n254 = property on="Incoming Water Temperature (2)" class="DigNum (strict)"("Visible"=w338) -> ()  [unwired: 2 in, 2 out]
            n255 = property on="Flow Rate (GPM 3)" class="DigNum (strict)"("Visible"=w337) -> ()  [unwired: 2 in, 2 out]
            n256 = property on="Flow Rate (GPM 2)" class="DigNum (strict)"("Visible"=w338) -> ()  [unwired: 2 in, 2 out]
          }
          frame "Two Pre-Draws" {
            w343 = FALSE ("Visible")
            n257 = case shown="True" w342 {
              frame False {
                w345 = TRUE ("Visible")
                n258 = property on="Description 1" class="Str"("Visible"=w345) -> ()  [unwired: 2 in, 2 out]
                n259 = property on="Total Gallons (1)" class="DigNum (strict)"("Visible"=w345) -> ()  [unwired: 2 in, 2 out]
                n260 = property on="Incoming Water Temperature (1)" class="DigNum (strict)"("Visible"=w345) -> ()  [unwired: 2 in, 2 out]
                n261 = property on="Flow Rate (GPM 1)" class="DigNum (strict)"("Visible"=w345) -> ()  [unwired: 2 in, 2 out]
              }
              frame True {
                w346 = FALSE ("Visible")
                n262 = property on="Description 1" class="Str"("Visible"=w346) -> ()  [unwired: 2 in, 2 out]
                n263 = property on="Total Gallons (1)" class="DigNum (strict)"("Visible"=w346) -> ()  [unwired: 2 in, 2 out]
                n264 = property on="Incoming Water Temperature (1)" class="DigNum (strict)"("Visible"=w346) -> ()  [unwired: 2 in, 2 out]
                n265 = property on="Flow Rate (GPM 1)" class="DigNum (strict)"("Visible"=w346) -> ()  [unwired: 2 in, 2 out]
              }
            }
            n266 = case shown="True" w344 {
              frame False {
                w347 = TRUE ("Visible")
                n267 = property on="Description 2" class="Str"("Visible"=w347) -> ()  [unwired: 2 in, 2 out]
                n268 = property on="Total Gallons (2)" class="DigNum (strict)"("Visible"=w347) -> ()  [unwired: 2 in, 2 out]
                n269 = property on="Incoming Water Temperature (2)" class="DigNum (strict)"("Visible"=w347) -> ()  [unwired: 2 in, 2 out]
                n270 = property on="Flow Rate (GPM 2)" class="DigNum (strict)"("Visible"=w347) -> ()  [unwired: 2 in, 2 out]
              }
              frame True {
                w348 = FALSE ("Visible")
                n271 = property on="Description 2" class="Str"("Visible"=w348) -> ()  [unwired: 2 in, 2 out]
                n272 = property on="Total Gallons (2)" class="DigNum (strict)"("Visible"=w348) -> ()  [unwired: 2 in, 2 out]
                n273 = property on="Incoming Water Temperature (2)" class="DigNum (strict)"("Visible"=w348) -> ()  [unwired: 2 in, 2 out]
                n274 = property on="Flow Rate (GPM 2)" class="DigNum (strict)"("Visible"=w348) -> ()  [unwired: 2 in, 2 out]
              }
            }
            n275 = property on="Description 3" class="Str"("Visible"=w343) -> ()  [unwired: 2 in, 2 out]
            n276 = property on="Total Gallons (3)" class="DigNum (strict)"("Visible"=w343) -> ()  [unwired: 2 in, 2 out]
            n277 = property on="Incoming Water Temperature (3)" class="DigNum (strict)"("Visible"=w343) -> ()  [unwired: 2 in, 2 out]
            n278 = property on="Flow Rate (GPM 3)" class="DigNum (strict)"("Visible"=w343) -> ()  [unwired: 2 in, 2 out]
          }
          frame "Three Pre-Draws" {
            n279 = case shown="True" w351 {
              frame False {
                w356 = TRUE ("Visible")
                n280 = property on="Description 3" class="Str"("Visible"=w356) -> ()  [unwired: 2 in, 2 out]
                n281 = property on="Total Gallons (3)" class="DigNum (strict)"("Visible"=w356) -> ()  [unwired: 2 in, 2 out]
                n282 = property on="Incoming Water Temperature (3)" class="DigNum (strict)"("Visible"=w356) -> ()  [unwired: 2 in, 2 out]
                n283 = property on="Flow Rate (GPM 3)" class="DigNum (strict)"("Visible"=w356) -> ()  [unwired: 2 in, 2 out]
              }
              frame True {
                w357 = FALSE ("Visible")
                n284 = property on="Description 3" class="Str"("Visible"=w357) -> ()  [unwired: 2 in, 2 out]
                n285 = property on="Total Gallons (3)" class="DigNum (strict)"("Visible"=w357) -> ()  [unwired: 2 in, 2 out]
                n286 = property on="Incoming Water Temperature (3)" class="DigNum (strict)"("Visible"=w357) -> ()  [unwired: 2 in, 2 out]
                n287 = property on="Flow Rate (GPM 3)" class="DigNum (strict)"("Visible"=w357) -> ()  [unwired: 2 in, 2 out]
              }
            }
            n288 = case shown="True" w350 {
              frame False {
                w354 = TRUE ("Visible")
                n289 = property on="Description 1" class="Str"("Visible"=w354) -> ()  [unwired: 2 in, 2 out]
                n290 = property on="Total Gallons (1)" class="DigNum (strict)"("Visible"=w354) -> ()  [unwired: 2 in, 2 out]
                n291 = property on="Incoming Water Temperature (1)" class="DigNum (strict)"("Visible"=w354) -> ()  [unwired: 2 in, 2 out]
                n292 = property on="Flow Rate (GPM 1)" class="DigNum (strict)"("Visible"=w354) -> ()  [unwired: 2 in, 2 out]
              }
              frame True {
                w355 = FALSE ("Visible")
                n293 = property on="Description 1" class="Str"("Visible"=w355) -> ()  [unwired: 2 in, 2 out]
                n294 = property on="Total Gallons (1)" class="DigNum (strict)"("Visible"=w355) -> ()  [unwired: 2 in, 2 out]
                n295 = property on="Incoming Water Temperature (1)" class="DigNum (strict)"("Visible"=w355) -> ()  [unwired: 2 in, 2 out]
                n296 = property on="Flow Rate (GPM 1)" class="DigNum (strict)"("Visible"=w355) -> ()  [unwired: 2 in, 2 out]
              }
            }
            n297 = case shown="True" w349 {
              frame False {
                w352 = TRUE ("Visible")
                n298 = property on="Description 2" class="Str"("Visible"=w352) -> ()  [unwired: 2 in, 2 out]
                n299 = property on="Total Gallons (2)" class="DigNum (strict)"("Visible"=w352) -> ()  [unwired: 2 in, 2 out]
                n300 = property on="Incoming Water Temperature (2)" class="DigNum (strict)"("Visible"=w352) -> ()  [unwired: 2 in, 2 out]
                n301 = property on="Flow Rate (GPM 2)" class="DigNum (strict)"("Visible"=w352) -> ()  [unwired: 2 in, 2 out]
              }
              frame True {
                w353 = FALSE ("Visible")
                n302 = property on="Description 2" class="Str"("Visible"=w353) -> ()  [unwired: 2 in, 2 out]
                n303 = property on="Total Gallons (2)" class="DigNum (strict)"("Visible"=w353) -> ()  [unwired: 2 in, 2 out]
                n304 = property on="Incoming Water Temperature (2)" class="DigNum (strict)"("Visible"=w353) -> ()  [unwired: 2 in, 2 out]
                n305 = property on="Flow Rate (GPM 2)" class="DigNum (strict)"("Visible"=w353) -> ()  [unwired: 2 in, 2 out]
              }
            }
          }
        }
        n306 = call <vilib>:"Add State(s) to Queue__jki_lib_state_machine.vi"("State(s) in (\"\")"=w331) -> ("States Out"=w330:string)  [unwired: 14 in]
      }
      frame "Read Dispense Time" {
        n307 = Unbundle By Name(w364) -> ("Pattern Setup"=w368:dbl[][], "Any Heat (1)"=w361:bool, "Any Heat (2)"=w360:bool, "Any Heat (3)"=w359:bool)
        n308 = Index Array(array=w368, index (col)=2) -> (element=w365:dbl[])  [unwired: 1 in]
        n309 = Index Array(array=w368, index (col)=0 ("disabled index (col)")) -> (element=w367:dbl[])  [unwired: 1 in]
        n310 = Index Array(array=w368, index (col)=1) -> (element=w366:dbl[])  [unwired: 1 in]
        n311 = for {
          tunnel: w367 -> [w380] mode=indexing
          tunnel: w366 -> [w379] mode=indexing
          tunnel: w365 -> [w376] mode=indexing
          tunnel: [w375] -> w362 mode=indexing
          n312 = expression code="x*60"(w379) -> (w377:dbl)
          n313 = expression code="x*3600"(w380) -> (w378:dbl)
          n314 = Compound Arithmetic op=ADD(w378, w377, w376) -> (w375:dbl)
        }
        n315 = Build Array(w361, w360, w359) -> (w358:bool[])
        n316 = Bundle By Name(cluster=w364, "Dispense Times"=w362, "Pre-Draw Until?"=w358) -> (w363:T24)
        n317 = call <vilib>:"Add State(s) to Queue__jki_lib_state_machine.vi"("State(s) in (\"\")"=w374) -> ("States Out"=w373:string)  [unwired: 14 in]
      }
      frame "Read Remaining" {
        # "Get the remaining dispense patterns"
        n318 = Unbundle By Name(w389) -> ("Pattern Setup"=w384:dbl[][], "PreDraw Enum"=w381:T21)
        n319 = Index Array(array=w384, index (col)=3 ("disabled index (col)")) -> (element=w387:dbl[])  [unwired: 1 in]
        n320 = Index Array(array=w384, index (col)=4 ("disabled index (col)")) -> (element=w383:dbl[])  [unwired: 1 in]
        n321 = Index Array(array=w384, index (col)=5 ("disabled index (col)")) -> (element=w382:dbl[])  [unwired: 1 in]
        n322 = Bundle By Name(cluster=w389, "Core HEWH Data Input.Test Patten Setup.Total Gallons Schedule"=w387, "Flow Rate Schedule"=w383, "Incoming Water Temperature"=w382, "24 Hour PreDraw"=w381) -> (w388:T24)
        n323 = call <vilib>:"Add State(s) to Queue__jki_lib_state_machine.vi"("State(s) in (\"\")"=w393) -> ("States Out"=w392:string)  [unwired: 14 in]
      }
      frame "PreDraw Pattern" {
        n324 = Unbundle By Name(w407) -> ("PreDraw Enum"=w406:T21, "PreDraw Pattern"=w394)
        n325 = case shown="\"One Pre- Draws\"" w406 {
          tunnel: [dbl[][] [] w412 w426 w440] -> w405
          tunnel: "Total Gallons (1)" -> [_ w417 w425 w439]
          tunnel: "Flow Rate (GPM 1)" -> [_ w416 w424 w438]
          tunnel: "Incoming Water Temperature (1)" -> [_ w415 w423 w437]
          tunnel: "Total Gallons (2)" -> [_ _ w422 w436]
          tunnel: "Flow Rate (GPM 2)" -> [_ _ w421 w435]
          tunnel: "Incoming Water Temperature (2)" -> [_ _ w420 w434]
          tunnel: "Total Gallons (3)" -> [_ _ _ w433]
          tunnel: "Flow Rate (GPM 3)" -> [_ _ _ w432]
          tunnel: "Incoming Water Temperature (3)" -> [_ _ _ w431]
          tunnel: w394 -> [_ w413 w427 w441]
          frame "Zero Pre-Draws", Default {
          }
          frame "One Pre- Draws" {
            n326 = Build Array(w417, w416, w415) -> (w414:dbl[])
            n327 = Build Array (concatenate)(w413, w414) -> (w412:dbl[][])
          }
          frame "Two Pre-Draws" {
            n328 = Build Array(w422, w421, w420) -> (w418:dbl[])
            n329 = Build Array(w425, w424, w423) -> (w419:dbl[])
            n330 = Build Array (concatenate)(w427, w419, w418) -> (w426:dbl[][])
          }
          frame "Three Pre-Draws" {
            n331 = Build Array(w439, w438, w437) -> (w430:dbl[])
            n332 = Build Array(w436, w435, w434) -> (w429:dbl[])
            n333 = Build Array(w433, w432, w431) -> (w428:dbl[])
            n334 = Build Array (concatenate)(w441, w430, w429, w428) -> (w440:dbl[][])
          }
        }
        "PreDraw\nPattern" <- w405
        n335 = Bundle By Name(cluster=w407, "PreDraw Pattern"=w405) -> (w408:T24)
        n336 = call <vilib>:"Add State(s) to Queue__jki_lib_state_machine.vi"("State(s) in (\"\")"=w409) -> ("States Out"=w410:string)  [unwired: 14 in]
      }
      frame "Display and Exit" {
        n337 = Unbundle By Name(w448) -> ("Core HEWH Data Input"=→"Core HEWH Data Input Out":T1, "PreDraw Pattern"=w443)
        n338 = Array Size(array=w443) -> (size(s)=w447:i32)
        n339 = Index Array(array=w447, index=0) -> (element=w445)
        n340 = Equal To 0?(x=w445) -> (x = 0?=→"Display and Exit":bool)
        n341 = call <vilib>:"Add State(s) to Queue__jki_lib_state_machine.vi"("State(s) in (\"\")"=w450) -> ("States Out"=w451:string)  [unwired: 14 in]
      }
    }
  }
  "error out" <- w1
